vi "DIsco_Main.vi"() -> ()   [LabVIEW 2017]
doc: "DIsco V1.X\n\nDeveloped by Luke P Frash\nLos Alamos National Laboratory"
uses:
  DIsco_Subs.llb/DIsco_Globals.vi
panel:
  out "COM":bool=TRUE
  out "WARN":bool=TRUE
  out "LNK":bool
  out "INIT":bool
  out "AUX":bool
  out "CALL":bool
  in  "Enable Data Saving":bool=TRUE caption="Enable"
  in  "Filename":path=path "C:/ProgramData/Sys_DIsc.lvm"
  out "Date":string
  in  "HistData Empty":bool
  in  "HistData Clear":bool
  out "Recorded Data":string[][](table)
  in  "stop":bool
  in  "Tab Control":enum32{"Valve Positions", "Valve Control Mode"}(tab)
  in  "Valve 4":bool
  in  "Valve 3":bool
  in  "Valve 2":bool
  in  "Valve":bool
  out "VI 1":bool
  out "VI 2":bool
  out "VI 3":bool
  out "VI 4":bool
  in  "Valve 8":bool
  in  "Valve 7":bool
  in  "Valve 6":bool
  in  "Valve 5":bool
  out "VI 5":bool
  out "VI 6":bool
  out "VI 7":bool
  out "VI 8":bool
  in  "SetValves":bool
  in  "Valve 13":bool
  in  "Valve 14":bool
  in  "Valve 15":bool
  in  "Valve 16":bool
  out "VI 13":bool
  out "VI 14":bool
  out "VI 15":bool
  out "VI 16":bool
  in  "Valve 9":bool
  in  "Valve 10":bool
  in  "Valve 11":bool
  in  "Valve 12":bool
  out "VI 9":bool
  out "VI 10":bool
  out "VI 11":bool
  out "VI 12":bool
  in  "SetValves 2":bool
  out "Valve R I":bool
  in  "Set Valve Control":bool
  out "ERR":bool=TRUE
  out "Program":bool
  in  "Track Pump Index":bool=TRUE
  out "F Active":dbl
  out "P Active":dbl
  out "Name of Selected Pump":string
  in  "RenamePump":bool
  in  "Rename":string
  out "CF Ind":bool
  out "CP Ind":bool
  out "CCP Ind":bool
  out "CCF Ind":bool
  in  "CCF":bool
  in  "CCP":bool
  in  "Remote":bool
  in  "Control ID":i32 min=0
  out "Status":string[](array[string])
  out "Pump Type":string
  out "Call ID":i32
  in  "Zero Pres":bool
  out "Letter":string
  in  "Pump Index":i32 min=0 max=4
  out "V Active":dbl
  out "Vol %":u8(slide) scale=0.0..100.0
  in  "Stop":bool
  in  "Run":bool
  in  "CP":bool
  in  "CF":bool
  in  "Pressure Setpoint":dbl min=0.0
  in  "Flow Setpoint":dbl
  in  "SetPress":bool
  in  "SetFlow":bool
  in  "Stop Pumps":bool
  out "Plot1 3":cluster{"X":dbl[], "Y":dbl[]}[](graph) caption="XY Graph"
  in  "X":string="Time"
  in  "Ref":string="log(0)"
  in  "Y6":string
  in  "Y5":string
  in  "Y4":string
  in  "Y3":string
  in  "Y2":string
  in  "Y1":string
  in  "Max_Y 3":dbl=68947.5729
  in  "Min_Y 3":dbl
  in  "Num Points 3":i32=100 min=2 max=10000 step=1
  in  "Max Log":dbl=30.0 min=1e-08 max=1000.0
  in  "Min Log":dbl=1e-06 min=1e-08 max=1000.0
  out "Pump Matrix":string[][](table)
  in  "Tab Control 2":T1(tab)
  in  "Program Edit Table":string[][](table)
  in  "Remove":bool
  in  "AddIt":bool
  in  "Program Selector":i32 min=-1 max=13
  in  "Routine Name":string caption="Program Editor / Importer"
  out "Meaning":string="cSUB PROGRAM : Initiates the pre-set program of NAME."
  out "Active Routine":string="RemoteStartup"
  out "Step":i32
  in  "Set Program":bool
  in  "Reset":bool
  in  "Run Program":bool
  in  "Import CSV":bool
  in  "Export":bool
  out "Countdown":dbl format="%#.1f"
  in  "Pump Index 2":i32 caption="Pump Index" min=0 max=1
  in  "Command":string
  in  "Manual\nExecute":bool
  out "Previous Serial Reply":string
  in  "Append":string caption="Append (eg 13.37)"
  in  "Browse":i32=28 min=0
  out "Description":string
  out "Previous Command":string
  in  "Add Var":bool
  in  "Set Var":bool
  in  "Input Variable (Name=Function)":string
  out "Table Control":string[][](table)
  in  "Add V Index":i32 min=0
  out "Var N":string
  out "Var V":dbl
  in  "E_Add":bool
  out "External Data":dbl[][](array[numeric])
  in  "Import":bool
  in  "External File Path":path=path "C:/Users/299494/Documents/Research/Engineering Design/Programs/DIsco_v1.0/Test Data/Sys_ExtD.lvm"
  in  "E_Col_Name":string
  in  "E_Col_Index":i32
  in  "ExtData Clear":bool
  out "Prog Fetch":i32
  out "Prev Select":i32
  in  "Log Commands":bool=TRUE
  in  "Ask_Auto":bool=TRUE
  in  "Stop Pumps on Exit":bool=TRUE
  in  "Data Call Rate":dbl=1.0 min=0.0001 max=2.0
  in  "Start Time":dbl caption="Reference Date (Time Zero)" format="%#_8g"
  out "Call Execution Time (ms)":u32
  out "Scaling Relationship 3":string="Scaling Factor: 2000*log(WF**-(F+Res))+30000"
  out "Fetch":i32=-1
  out "Heirarchy":string
  out "Passing String":string
  out "Program Errors":string
  out "Running Program":string[][](table)
  out "Brow":i32=28
  out "EXIT":bool
  out "Remote Indicator":bool caption="R/I"
  # "*Units: Min, Days, kPa, mL/min, mL"
  # "Select Pump"
  # "Index"
  # "Letter"
  # "Type"
  # "Setpoint"
  # "Actual Value"
  # "Pump Name"
  # "Pressure (kPa)"
  # "Flow Rate (mL/min)"
  # "Volume (mL)"
  # "Pump Status"
  # "Valve Control"
  # "1"
  # "2"
  # "3"
  # "4"
  # "5"
  # "6"
  # "7"
  # "8"
  # "1"
  # "2"
  # "3"
  # "4"
  # "5"
  # "6"
  # "7"
  # "8"
  # "Plot Settings"
  # "Linear"
  # "log"
  # "Max Linear"
  # "Min Linear"
  # "Max Log"
  # "Min Log"
  # "Points"
  # "Active Routine"
  # "(min)"
  # "Edit Routine"
  # "Selector"
  # "Pump Routine Name"
  # "Manual Command Entry"
  # "Reply to Manual Command"
  # "Input Variable"
  # "Name=[Function] or [Value]"
  # "eg: \"Var1=Var2^2-log(3)/exp(2.32)\""
  # "Add Variable to Data History"
  # "Index"
  # "Name"
  # "Value"
  # "Variable List"
  # "Select CSV Data File to Import"
  # "Add New Column to Data History"
  # "Name"
  # "Col."
  # "Remove All External Data"
  # "Selected External Data"
  # "Data Aquisition Settings"
  # "Hz"
  # "Days"
  # "General Settings"
  # "Log Program Commands"
  # "Ask for Automatic Pump Detection"
  # "Plot Scaling"
  # "Pump Program Parameters"
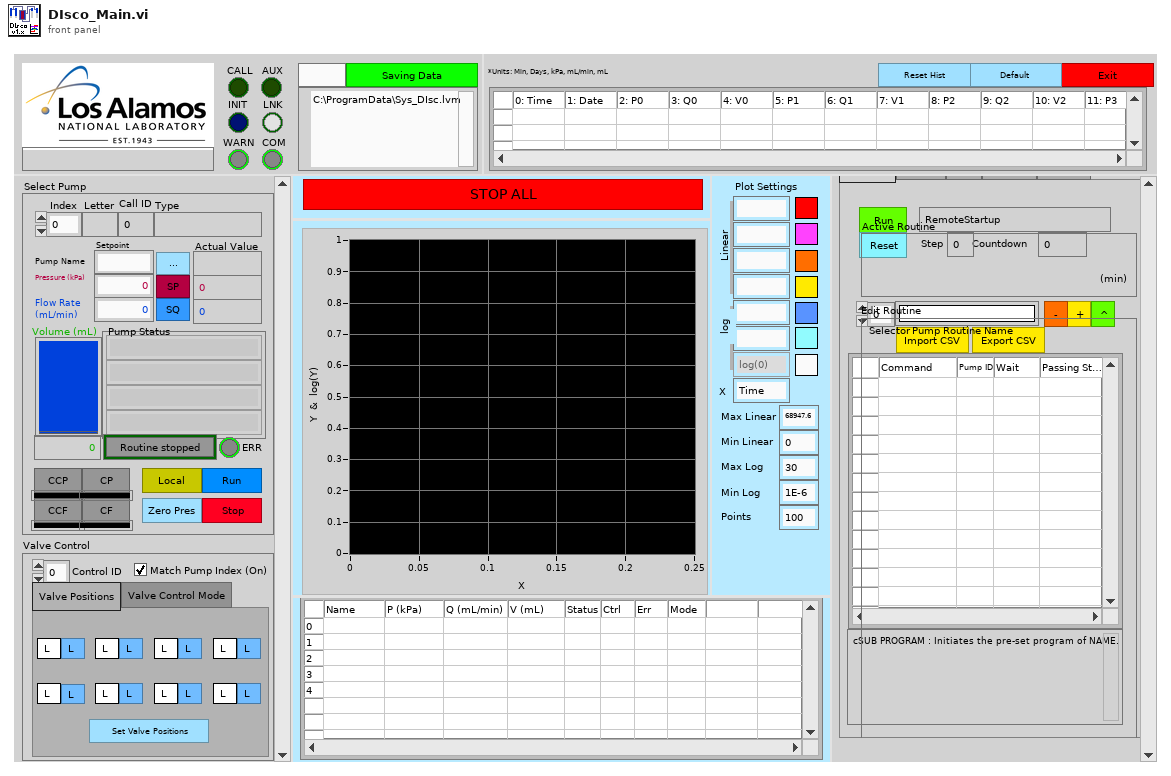
[diagram p1: front panel]
types:
  T1 = enum32{"Routines", "Manual", "Vars", "External", "Settings"}
  T2 = enum8{"Enabled", "Disabled", "Disabled and Grayed Out"}
  T3 = typedef "LVRowAndColumnTypeDef.ctl" = cluster{"Row":i32, "Column":i32}
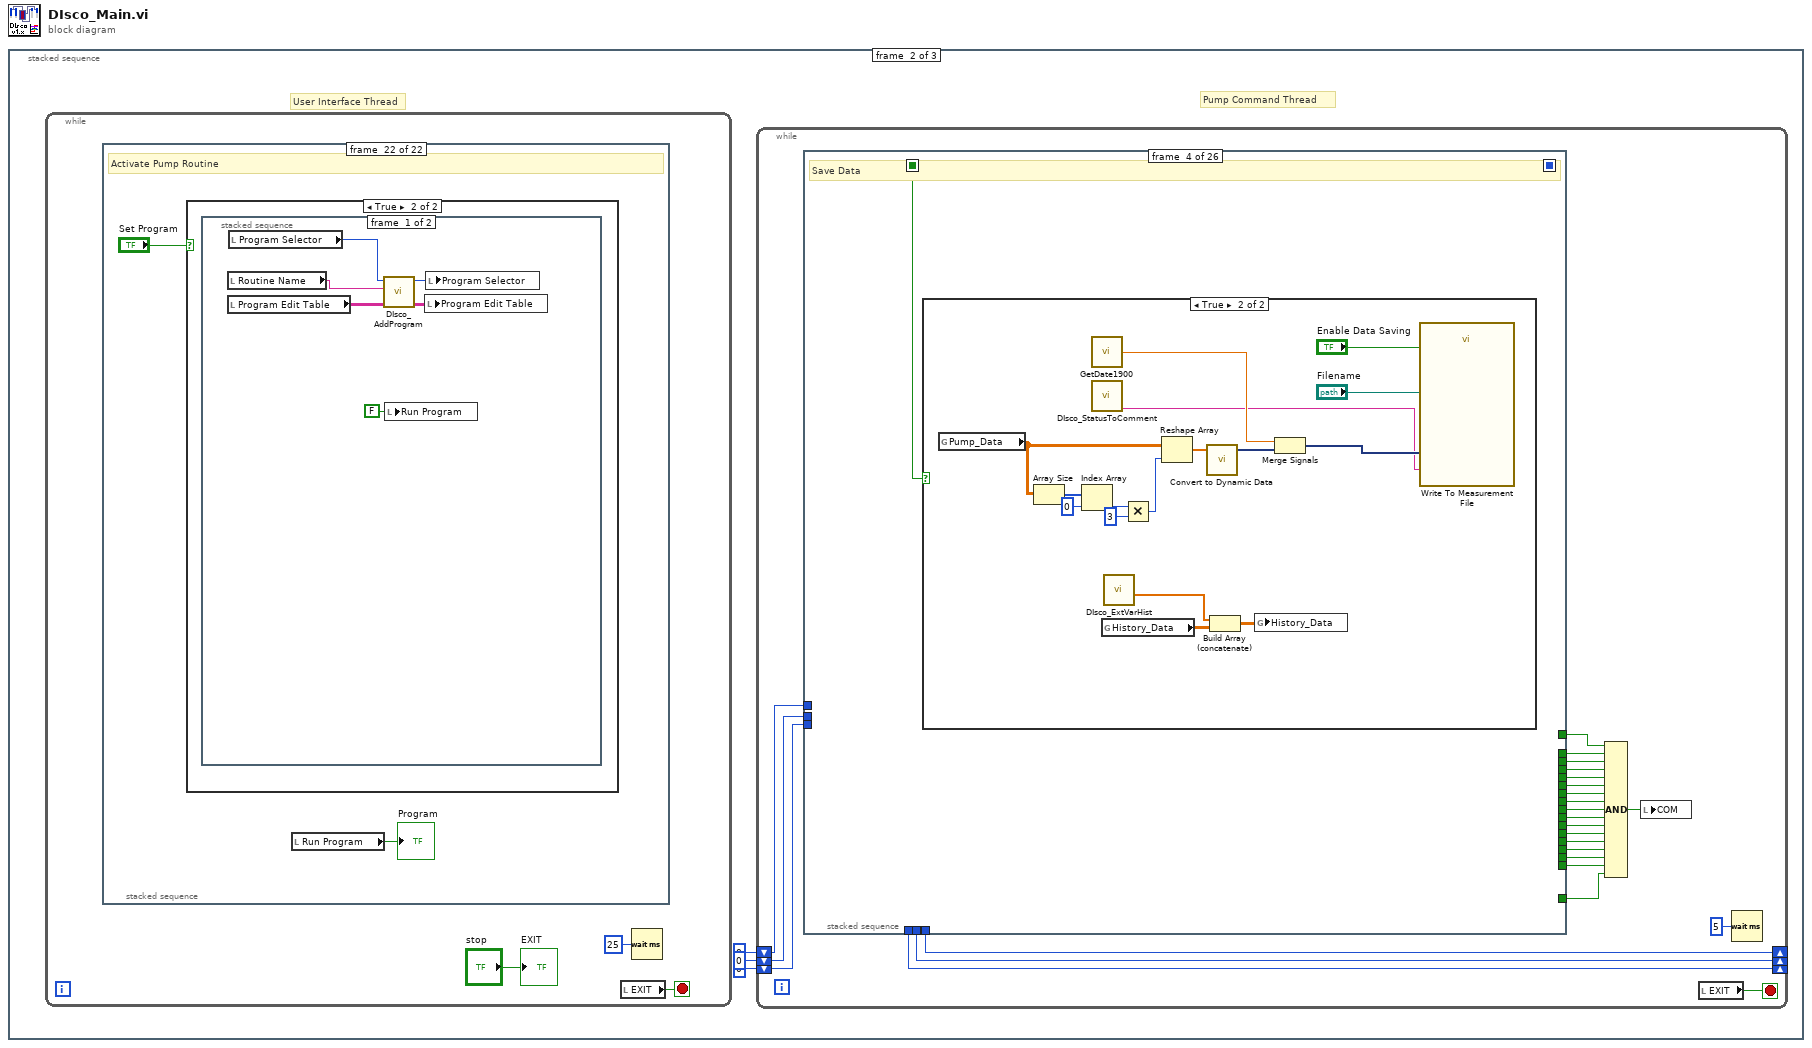
[diagram p0: block diagram]
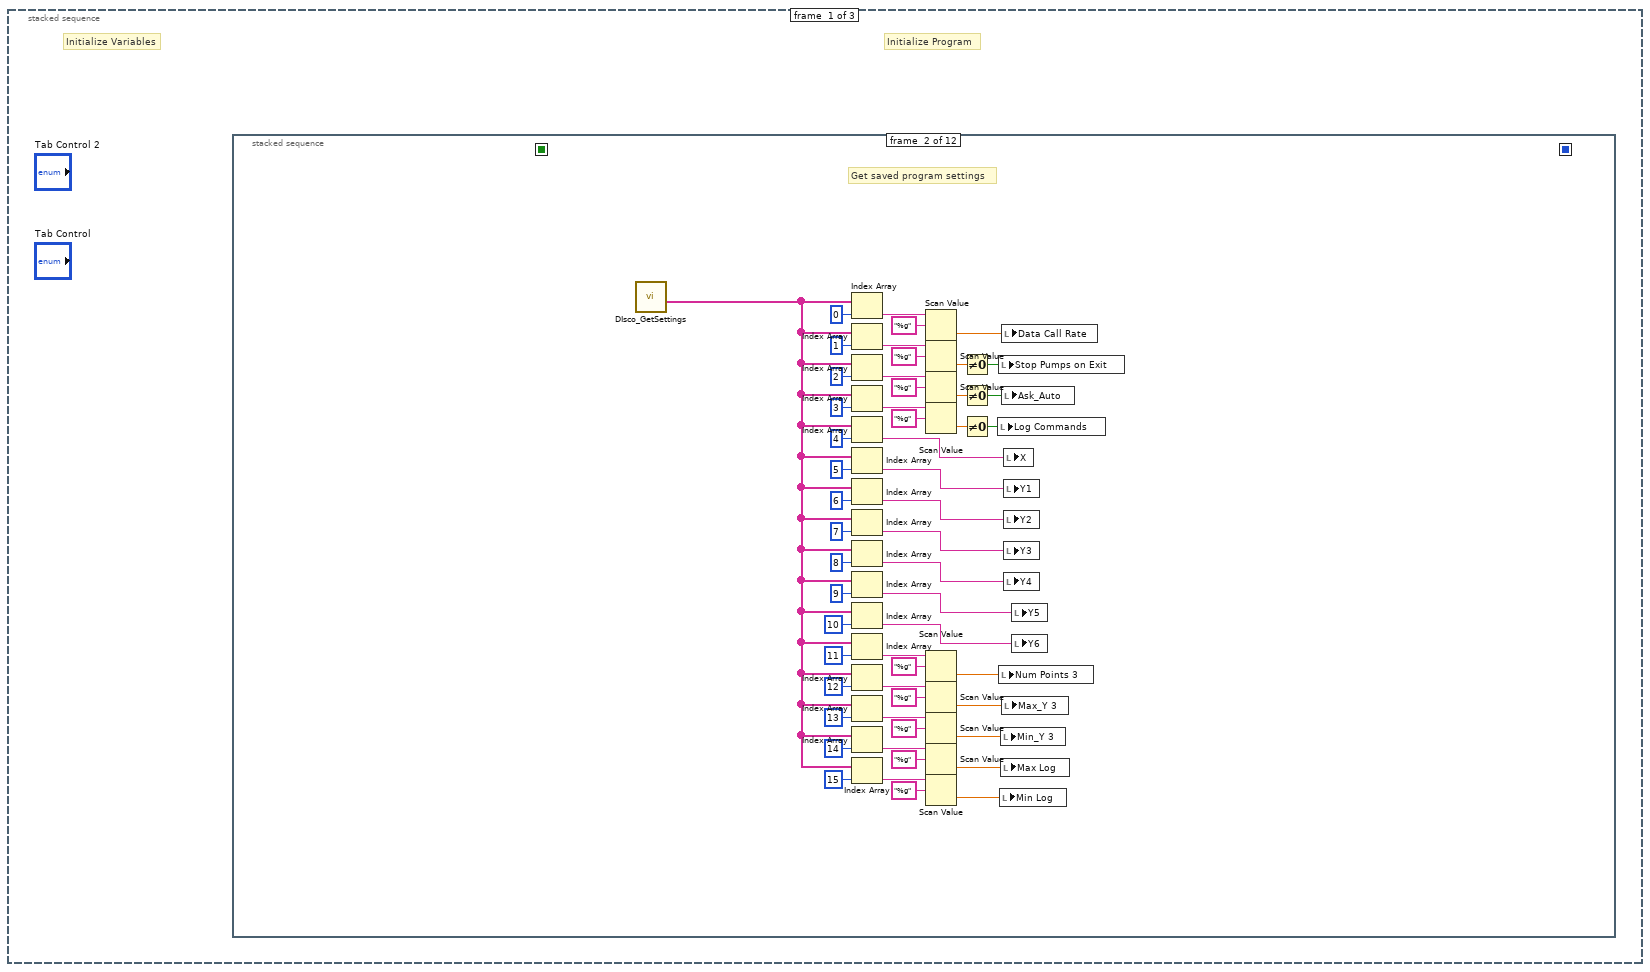
[diagram p2: hidden frame]
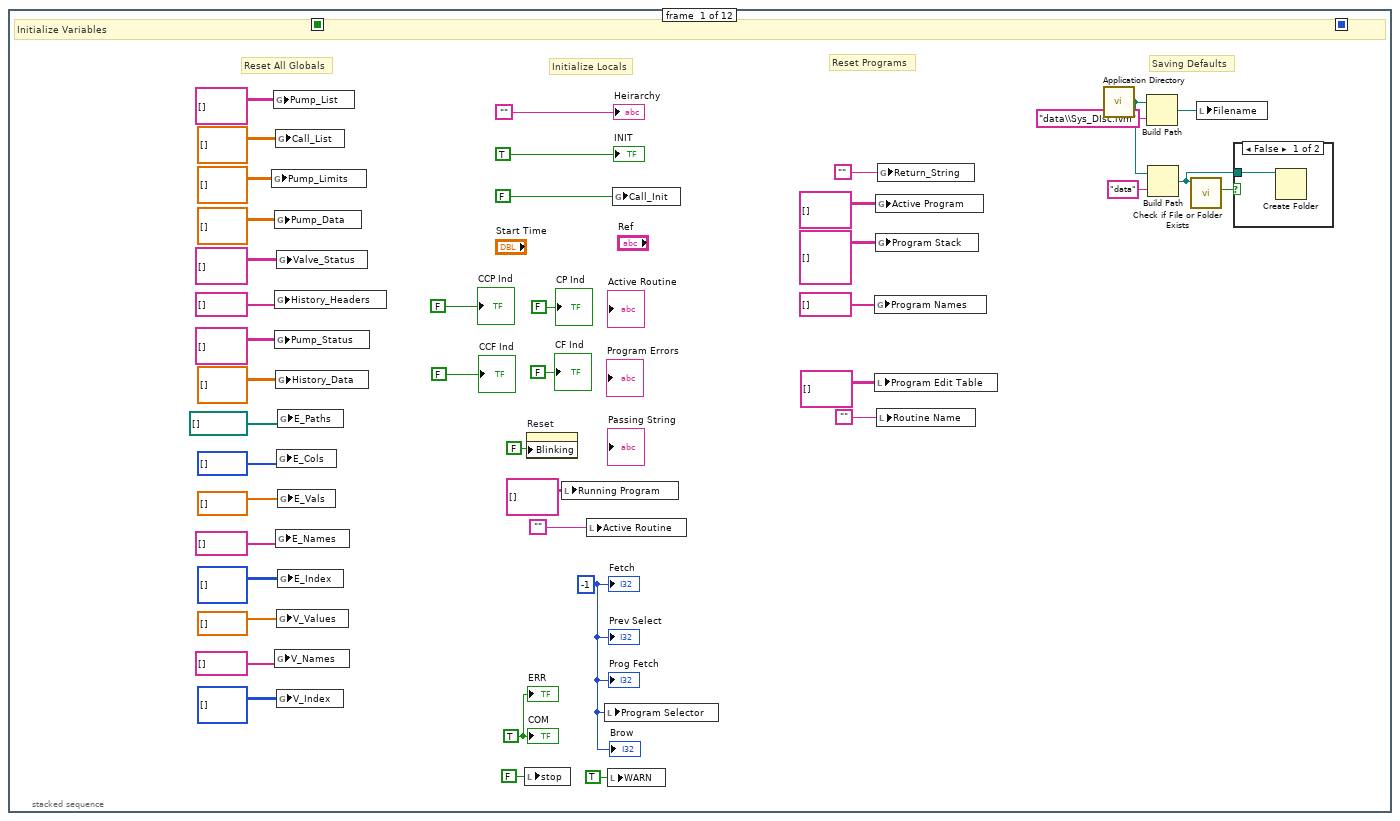
[diagram p3: hidden frame]
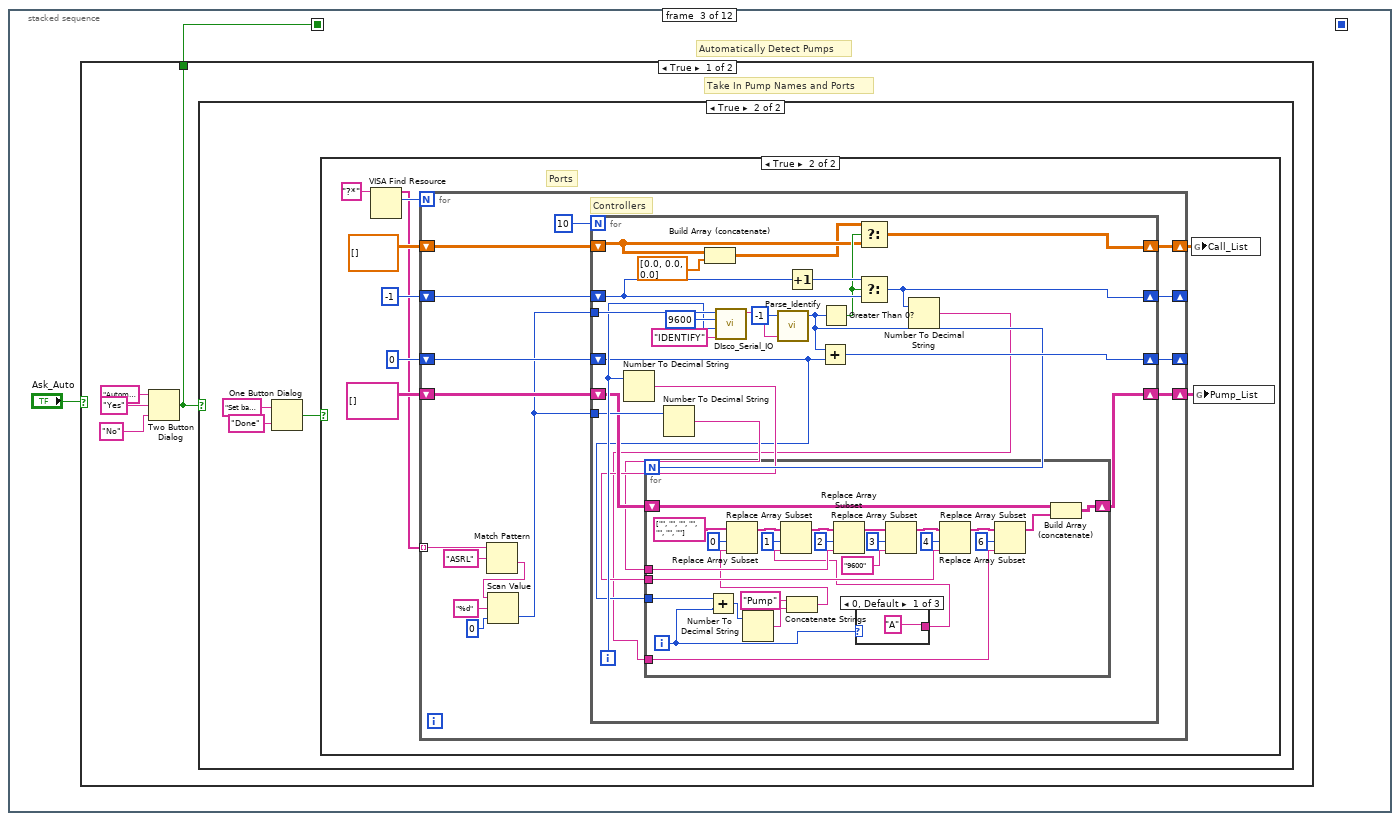
[diagram p5: hidden frame]
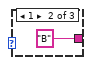
[diagram p8: hidden frame]
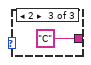
[diagram p9: hidden frame]
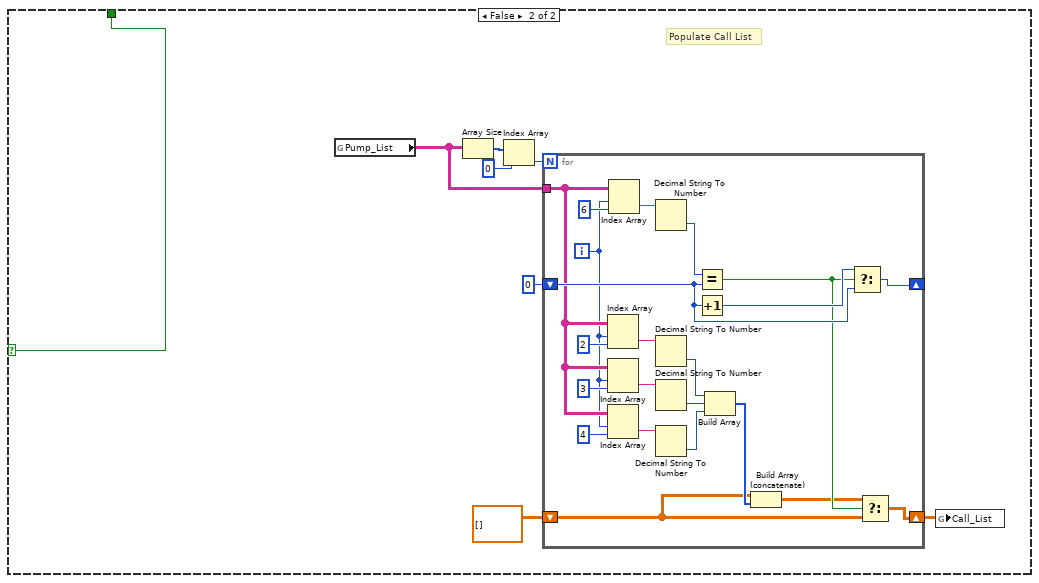
[diagram p10: hidden frame]
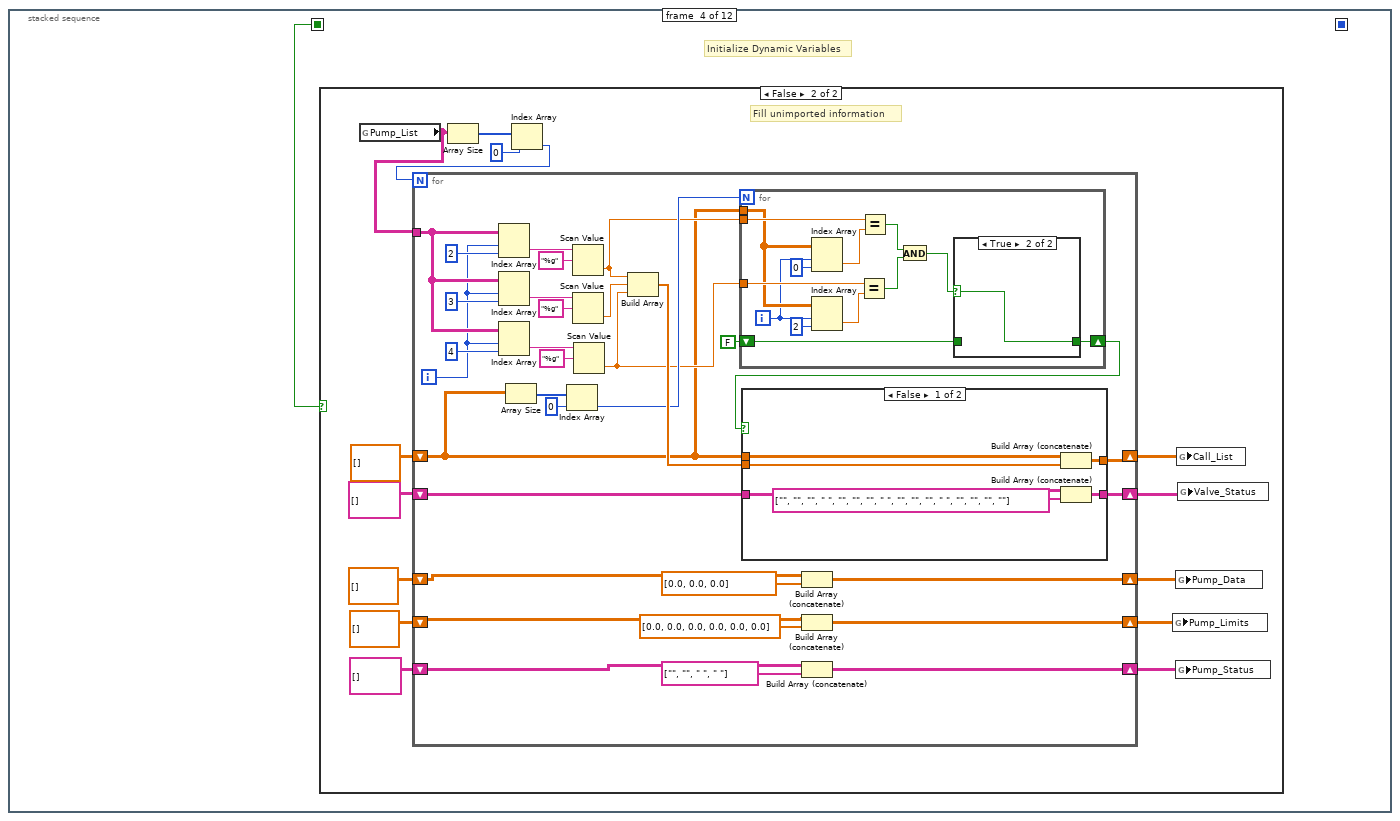
[diagram p11: hidden frame]
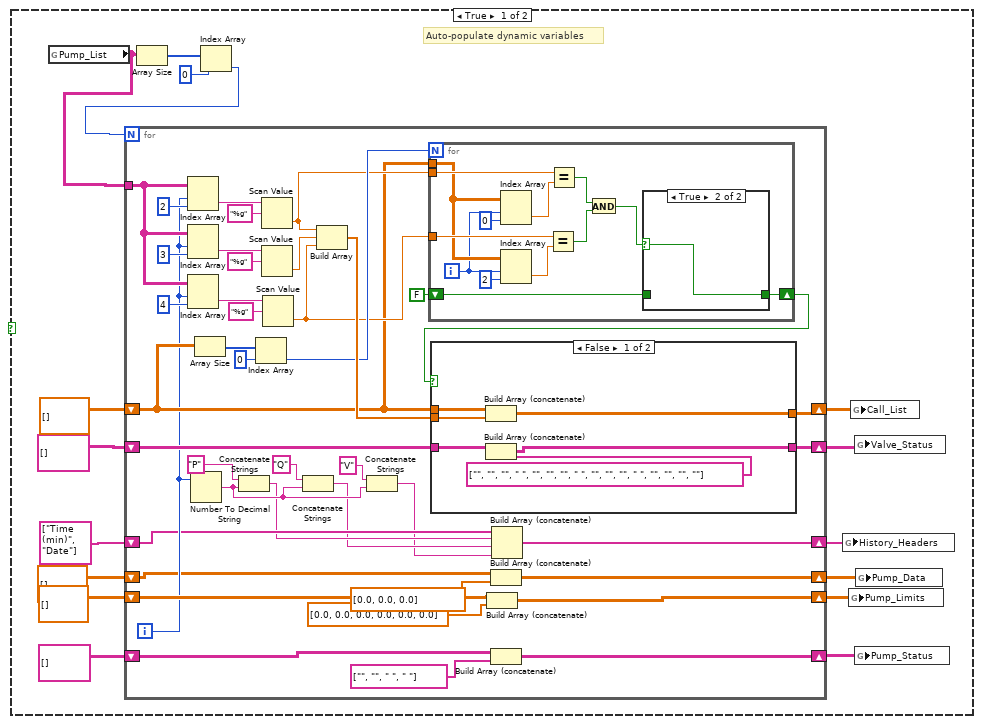
[diagram p12: hidden frame]
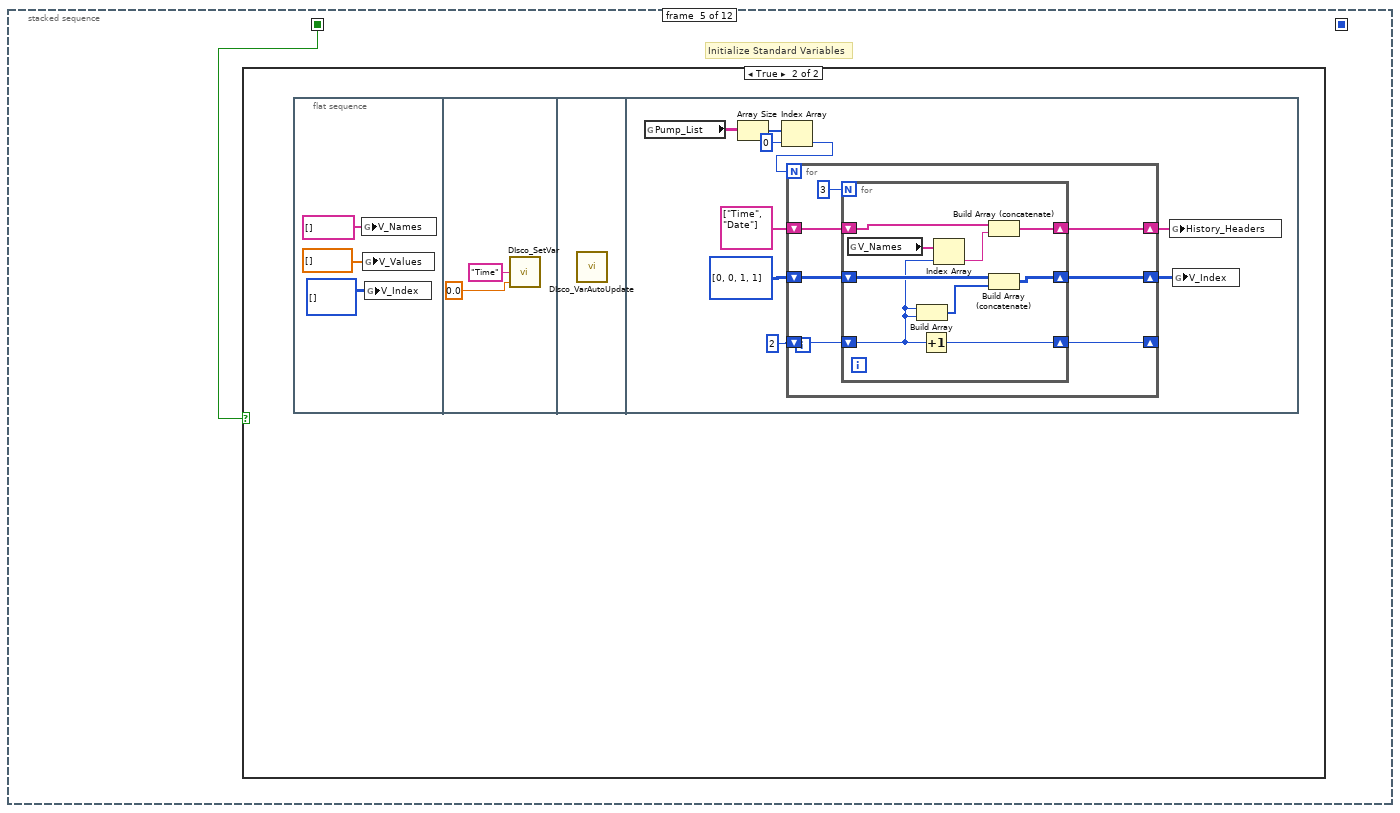
[diagram p17: hidden frame]
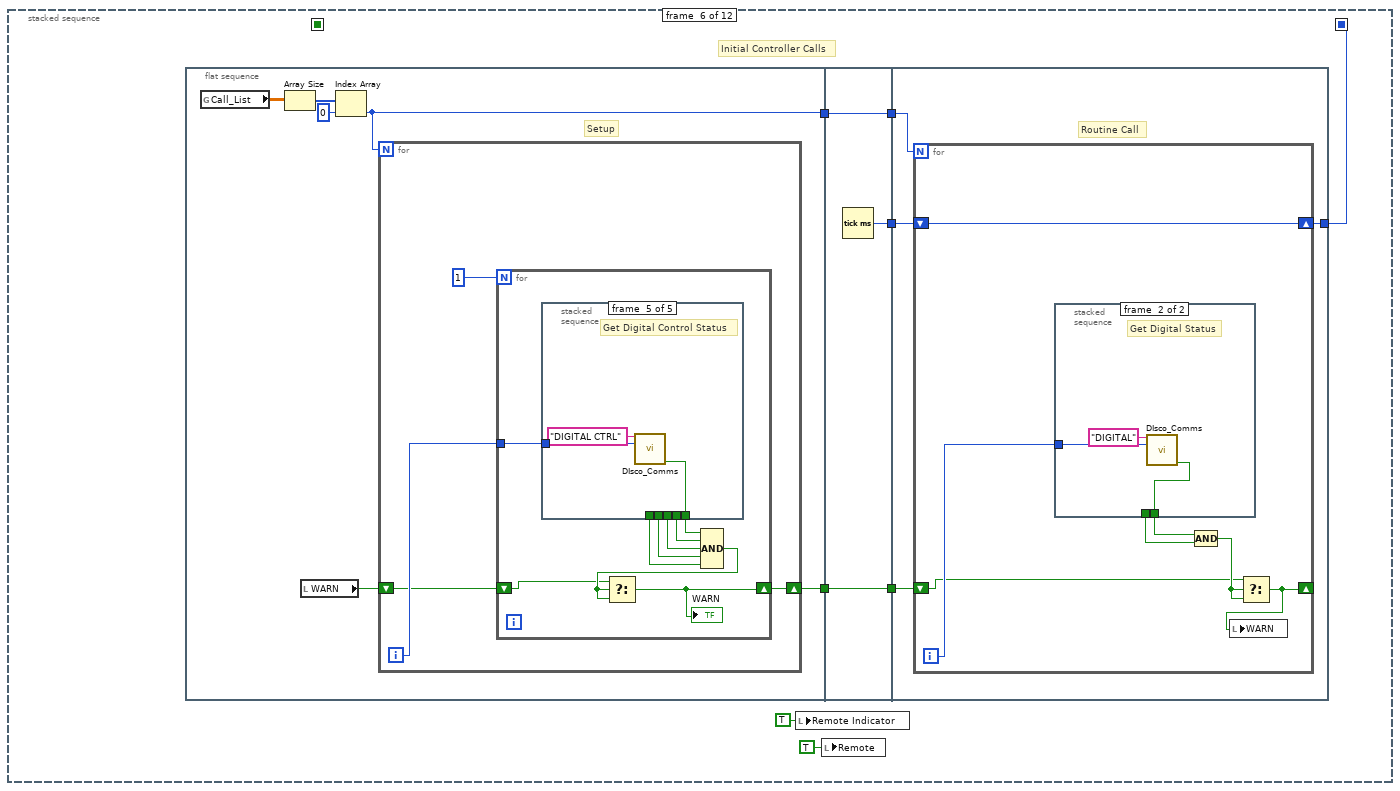
[diagram p19: hidden frame]
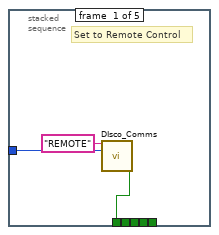
[diagram p20: hidden frame]
diagram:
  n1 = stacked-sequence {
    frame #0 {
      # "Initialize Variables"
      # "Initialize Program"
      n2 = stacked-sequence {
        seq-local: [_ _ w99 _ _ _ _ _ _ _ _ _] -> [_ _ _ w213 w365 _ w460 _ w492 _ _ _]
        seq-local: [_ _ _ _ _ w400 _ _ _ _ _ _] -> [_ _ _ _ _ _ w464 _ _ _ _ _]
        frame #0 {
          w1 = TRUE ("COM")
          w4 = -1 ("Fetch")
          # "Saving Defaults"
          # "Reset Programs"
          # "Initialize Locals"
          # "Reset All Globals"
          # "Initialize Variables"
          n3 = global write "DIsco_Globals.vi" "Pump_Limits"(dbl[][] [] ("Pump_Limits")) -> ()
          n4 = global write "DIsco_Globals.vi" "Pump_List"(string[][] [] ("Valve_Status")) -> ()
          n5 = global write "DIsco_Globals.vi" "Pump_Data"(dbl[][] [] ("Pump_Limits")) -> ()
          n6 = global write "DIsco_Globals.vi" "History_Headers"(string[] [] ("Valve_Status")) -> ()
          n7 = global write "DIsco_Globals.vi" "Pump_Status"(string[][] [] ("Valve_Status")) -> ()
          n8 = global write "DIsco_Globals.vi" "V_Names"(string[] [] ("Valve_Status")) -> ()
          n9 = global write "DIsco_Globals.vi" "Call_List"(dbl[][] [] ("Call_List")) -> ()
          n10 = global write "DIsco_Globals.vi" "History_Data"(dbl[][] [] ("History_Data")) -> ()
          n11 = global write "DIsco_Globals.vi" "E_Names"(string[] [] ("Valve_Status")) -> ()
          n12 = global write "DIsco_Globals.vi" "Valve_Status"(string[][] [] ("Valve_Status")) -> ()
          n13 = global write "DIsco_Globals.vi" "E_Cols"(i32[] [] ("E_Cols")) -> ()
          n14 = global write "DIsco_Globals.vi" "V_Values"(dbl[] [] ("History_Data")) -> ()
          n15 = global write "DIsco_Globals.vi" "V_Index"(i32[][] [] ("E_Cols")) -> ()
          n16 = global write "DIsco_Globals.vi" "E_Paths"(path[] [] ("E_Paths")) -> ()
          n17 = global write "DIsco_Globals.vi" "E_Vals"(dbl[] [] ("History_Data")) -> ()
          n18 = global write "DIsco_Globals.vi" "E_Index"(i32[][] [] ("E_Cols")) -> ()
          n19 = local write "stop"(FALSE ("stop")) -> ()
          n20 = property on="Reset" class="Bool (strict)"("Blinking"=FALSE) -> ()  [unwired: 2 in, 2 out]
          n21 = local write "Running Program"(string[][] [] ("Running Program")) -> ()
          n22 = local write "Active Routine"("") -> ()
          n23 = local write "Program Selector"(w4) -> ()
          n24 = local write "WARN"(TRUE ("WARN")) -> ()
          n25 = global write "DIsco_Globals.vi" "Call_Init"(FALSE ("Call_Init")) -> ()
          n26 = global write "DIsco_Globals.vi" "Program Names"(string[] [] ("Valve_Status")) -> ()
          n27 = local write "Program Edit Table"(string[][] [] ("Program Edit Table")) -> ()
          n28 = global write "DIsco_Globals.vi" "Active Program"(string[][] [] ("Valve_Status")) -> ()
          n29 = global write "DIsco_Globals.vi" "Program Stack"(string[][][] [] ("Valve_Status")) -> ()
          n30 = local write "Routine Name"("") -> ()
          n31 = global write "DIsco_Globals.vi" "Return_String"("") -> ()
          n32 = call <vilib>:"Application Directory.vi"() -> ("Application Directory"=w8:path)
          n33 = Build Path(base path=w8, name or relative path="data\\Sys_DIsc.lvm") -> (appended path=w22:path)
          n34 = Build Path(base path=w8, name or relative path="data") -> (appended path=w5:path)
          n35 = call <vilib>:"Check if File or Folder Exists.vi"("path"=w5) -> ("file or folder exists?"=w6:bool)  [unwired: 8 in, 2 out]
          n36 = local write "Filename"(w22) -> ()
          n37 = case shown="False" w6 {
            tunnel: w5 -> [w43 _]
            frame False {
              n38 = Create Folder(path (use dialog)=w43) -> ()  [unwired: 2 in, 3 out]
            }
            frame True {
            }
          }
          "INIT" <- TRUE ("INIT")
          "Heirarchy" <- ""
          "Fetch" <- w4
          "CP Ind" <- FALSE ("CCP Ind")
          "CF Ind" <- FALSE ("CCP Ind")
          "CCP Ind" <- FALSE ("CCP Ind")
          "CCF Ind" <- FALSE ("CCF Ind")
          "Prev Select" <- w4
          "Prog Fetch" <- w4
          "Brow" <- w4
          "COM" <- w1
          "ERR" <- w1
        }
        frame #1 {
          # "Get saved program settings"
          n39 = call "DIsco_GetSettings.vi"() -> ("General Settings"=w56:string[])  [unwired: 11 in]
          n40 = Index Array(array=w56, index=0) -> (element=w96:string)
          n41 = Index Array(array=w56, index=1) -> (element=w93:string)
          n42 = Index Array(array=w56, index=2) -> (element=w89:string)
          n43 = Index Array(array=w56, index=3) -> (element=w85:string)
          n44 = Index Array(array=w56, index=4) -> (element=w44:string)
          n45 = Index Array(array=w56, index=5) -> (element=w50:string)
          n46 = Index Array(array=w56, index=6) -> (element=w49:string)
          n47 = Index Array(array=w56, index=7) -> (element=w48:string)
          n48 = Index Array(array=w56, index=8) -> (element=w47:string)
          n49 = Index Array(array=w56, index=9) -> (element=w46:string)
          n50 = Index Array(array=w56, index=10) -> (element=w45:string)
          n51 = Index Array(array=w56, index=11) -> (element=w70:string)
          n52 = Index Array(array=w56, index=12) -> (element=w67:string)
          n53 = Index Array(array=w56, index=13) -> (element=w64:string)
          n54 = Index Array(array=w56, index=14) -> (element=w61:string)
          n55 = Index Array(array=w56, index=15) -> (element=w58:string)
          n56 = Scan Value(string=w96, format string="%g") -> (value=w82:dbl)  [unwired: 1 in, 1 out]
          n57 = Scan Value(string=w93, format string="%g") -> (value=w91:dbl)  [unwired: 1 in, 1 out]
          n58 = Scan Value(string=w89, format string="%g") -> (value=w87:dbl)  [unwired: 1 in, 1 out]
          n59 = Scan Value(string=w85, format string="%g") -> (value=w83:dbl)  [unwired: 1 in, 1 out]
          n60 = Scan Value(string=w70, format string="%g") -> (value=w55:dbl)  [unwired: 1 in, 1 out]
          n61 = Scan Value(string=w67, format string="%g") -> (value=w54:dbl)  [unwired: 1 in, 1 out]
          n62 = Scan Value(string=w64, format string="%g") -> (value=w53:dbl)  [unwired: 1 in, 1 out]
          n63 = Scan Value(string=w61, format string="%g") -> (value=w52:dbl)  [unwired: 1 in, 1 out]
          n64 = Scan Value(string=w58, format string="%g") -> (value=w51:dbl)  [unwired: 1 in, 1 out]
          n65 = Not Equal To 0?(x=w91) -> (x != 0?=w81:bool)
          n66 = Not Equal To 0?(x=w87) -> (x != 0?=w80:bool)
          n67 = Not Equal To 0?(x=w83) -> (x != 0?=w79:bool)
          n68 = local write "Log Commands"(w79) -> ()
          n69 = local write "Stop Pumps on Exit"(w81) -> ()
          n70 = local write "Num Points 3"(w55) -> ()
          n71 = local write "Min Log"(w51) -> ()
          n72 = local write "Min_Y 3"(w53) -> ()
          n73 = local write "Max Log"(w52) -> ()
          n74 = local write "Data Call Rate"(w82) -> ()
          n75 = local write "Ask_Auto"(w80) -> ()
          n76 = local write "Max_Y 3"(w54) -> ()
          n77 = local write "X"(w44) -> ()
          n78 = local write "Y1"(w50) -> ()
          n79 = local write "Y2"(w49) -> ()
          n80 = local write "Y3"(w48) -> ()
          n81 = local write "Y4"(w47) -> ()
          n82 = local write "Y5"(w46) -> ()
          n83 = local write "Y6"(w45) -> ()
        }
        frame #2 {
          # "Automatically Detect Pumps"
          n84 = case shown="True" "Ask_Auto" {
            selector: "Ask_Auto" -> [_ w185]
            tunnel: [w100 w185] -> w99
            frame True {
              # "Take In Pump Names and Ports"
              n85 = Two Button Dialog(message="Automatically detect attached pumps?", 1:"No" ("F button name (\"Cancel\")"), 2:"Yes" ("T button name (\"OK\")")) -> (T button?=w100:bool)
              n86 = case shown="True" w100 {
                frame False {
                }
                frame True {
                  n87 = One Button Dialog(message="Set baud rate on all controllers to 9600", button name ("OK")="Done") -> (true=w104:bool)
                  n88 = case shown="True" w104 {
                    frame False {
                    }
                    frame True {
                      # "Ports"
                      n89 = VISA Find Resource(11:"?*" ("expression (\"?*\")")) -> (2:w108:u32, 3:w107:string[])  [unwired: 2 in, 1 out]
                      n90 = for {
                        N: w108 -> [_]
                        shift-right: [w129] -> _
                        shift-left: 0 ("nCommand") -> [w130]
                        shift-right: [w126] -> _
                        shift-left: -1 ("nCommand") -> [w127]
                        shift-right: [w124] -> w112
                        shift-left: string[][] [] ("Pump_List") -> [w125]
                        shift-right: [w123] -> w110
                        shift-left: dbl[][] [] ("Call_List") -> [w122]
                        tunnel: w107 -> [w121] mode=indexing
                        # "Controllers"
                        n91 = Match Pattern(string=w121, regular expression="ASRL") -> (after substring=w119:string)  [unwired: 1 in, 3 out]
                        n92 = Scan Value(string=w119, format string="%d", default (0 dbl)=0) -> (value=w116:i32)  [unwired: 1 out]
                        n93 = for {
                          N: 10 -> [_]
                          shift-right: [w149] -> w129
                          shift-left: w130 -> [w139]
                          tunnel: w116 -> [w150]
                          shift-right: [w138] -> w126
                          shift-left: w127 -> [w147]
                          shift-right: [w142] -> w124
                          shift-left: w125 -> [w144]
                          tunnel: w116 -> [w145]
                          shift-right: [w133] -> w123
                          shift-left: w122 -> [w135]
                          i -> [w146]
                          n94 = Number To Decimal String(number=w146) -> (decimal integer string=w141:string)  [unwired: 1 in]
                          n95 = Number To Decimal String(number=w145) -> (decimal integer string=w140:string)  [unwired: 1 in]
                          n96 = Build Array (concatenate)(w135, dbl[] [0.0, 0.0, 0.0] ("Call_List")) -> (w134:dbl[][])
                          n97 = call "DIsco_Serial_IO.vi"("Pump Command"="IDENTIFY", "Controller ID"=w146, "Baud Rate"=9600, "Port"=w150) -> ("Reply"=w153:string)  [unwired: 6 in, 1 out]
                          n98 = call "Parse_Identify.vi"("Pump Info"=w153, "Call Index"=-1) -> ("Number of Pumps"=w143:i32)  [unwired: 1 in, 2 out]
                          n99 = Increment(x=w147) -> (x+1=w148:i32)
                          n100 = Add(x=w143, y=w139) -> (x+y=w149:i32)
                          n101 = Greater Than 0?(x=w143) -> (x > 0?=w136:bool)
                          n102 = Select(t=w134, s=w136, f=w135) -> (s? t:f=w133:dbl[][])
                          n103 = Select(t=w148, s=w136, f=w147) -> (s? t:f=w138:i32)
                          n104 = Number To Decimal String(number=w138) -> (decimal integer string=w137:string)  [unwired: 1 in]
                          n105 = for {
                            N: w143 -> [_]
                            shift-right: [w165] -> w142
                            shift-left: w144 -> [w166]
                            tunnel: w141 -> [w163]
                            tunnel: w140 -> [w162]
                            tunnel: w139 -> [w159]
                            tunnel: w137 -> [w155]
                            i -> [w154]
                            n106 = Add(x=w159, y=w154) -> (x+y=w158:i32)
                            n107 = Number To Decimal String(number=w158) -> (decimal integer string=w161:string)  [unwired: 1 in]
                            n108 = Concatenate Strings("Pump" ("string"), w161) -> (w157:string)
                            n109 = Replace Array Subset(array=string[] ["", "", "", "", "", "", ""] ("Array"), new element=w157, index=0) -> (w172:string[])
                            n110 = case shown="0, Default" w154 {
                              tunnel: ["A" ("new element/subarray") "B" ("new element/subarray") "C" ("new element/subarray")] -> w156
                              frame 0, Default {
                              }
                              frame 1 {
                              }
                              frame 2 {
                              }
                            }
                            n111 = Replace Array Subset(array=w172, new element=w156, index=1) -> (w171:string[])
                            n112 = Replace Array Subset(array=w171, new element=w162, index=2) -> (w170:string[])
                            n113 = Replace Array Subset(array=w170, new element="9600" ("new element/subarray"), index=3) -> (w169:string[])
                            n114 = Replace Array Subset(array=w169, new element=w163, index=4) -> (w168:string[])
                            n115 = Replace Array Subset(array=w168, new element=w155, index=6) -> (w167:string[])
                            n116 = Build Array (concatenate)(w166, w167) -> (w165:string[][])
                          }
                        }
                      }
                      n117 = global write "DIsco_Globals.vi" "Call_List"(w110) -> ()
                      n118 = global write "DIsco_Globals.vi" "Pump_List"(w112) -> ()
                    }
                  }
                }
              }
            }
            frame False {
              # "Populate Call List"
              n119 = global read "DIsco_Globals.vi" "Pump_List"() -> (w184:string[][])
              n120 = Array Size(array=w184) -> (size(s)=w188:i32[])
              n121 = Index Array(array=w188, index=0) -> (element=w186:i32)
              n122 = for {
                N: w186 -> [_]
                shift-right: [w191] -> w189
                shift-left: dbl[][] [] ("Call_List") -> [w192]
                tunnel: w184 -> [w203]
                shift-right: [w207] -> _
                shift-left: 0 ("index") -> [w208]
                i -> [w202]
                n123 = Index Array(array=w203, index (row)=w202, index (col)=2 ("disabled index (col)")) -> (element=w201:string)
                n124 = Index Array(array=w203, index (row)=w202, index (col)=3 ("disabled index (col)")) -> (element=w200:string)
                n125 = Index Array(array=w203, index (row)=w202, index (col)=4 ("disabled index (col)")) -> (element=w199:string)
                n126 = Index Array(array=w203, index (row)=w202, index (col)=6 ("disabled index (col)")) -> (element=w211:string)
                n127 = Decimal String To Number(string=w211) -> (number=w210:i32)  [unwired: 2 in, 1 out]
                n128 = Decimal String To Number(string=w201) -> (number=w198:i32)  [unwired: 2 in, 1 out]
                n129 = Decimal String To Number(string=w200) -> (number=w197:i32)  [unwired: 2 in, 1 out]
                n130 = Decimal String To Number(string=w199) -> (number=w196:i32)  [unwired: 2 in, 1 out]
                n131 = Equal?(x=w210, y=w208) -> (x = y?=w195:bool)
                n132 = Increment(x=w208) -> (x+1=w209:i32)
                n133 = Build Array(w198, w197, w196) -> (w194:i32[])
                n134 = Build Array (concatenate)(w192, w194) -> (w193:dbl[][])
                n135 = Select(t=w209, s=w195, f=w208) -> (s? t:f=w207:i32)
                n136 = Select(t=w193, s=w195, f=w192) -> (s? t:f=w191:dbl[][])
              }
              n137 = global write "DIsco_Globals.vi" "Call_List"(w189) -> ()
            }
          }
        }
        frame #3 {
          # "Initialize Dynamic Variables"
          n138 = case shown="False" w213 {
            frame True {
              # "Auto-populate dynamic variables"
              n139 = global read "DIsco_Globals.vi" "Pump_List"() -> (w219:string[][])
              n140 = Array Size(array=w219) -> (size(s)=w229:i32[])
              n141 = Index Array(array=w229, index=0) -> (element=w218:i32)
              n142 = for {
                N: w218 -> [_]
                shift-right: [w265] -> w226
                shift-left: dbl[][] [] ("Call_List") -> [w247]
                shift-right: [w266] -> w224
                shift-left: dbl[][] [] ("Call_List") -> [w267]
                tunnel: w219 -> [w248]
                shift-right: [w244] -> w222
                shift-left: string[][] [] ("Valve_Status") -> [w245]
                shift-right: [w256] -> w220
                shift-left: dbl[][] [] ("Call_List") -> [w241]
                shift-right: [w242] -> w216
                shift-left: string[] ["Time (min)", "Date"] ("Valve_Status") -> [w240]
                shift-right: [w230] -> w215
                shift-left: string[][] [] ("Valve_Status") -> [w231]
                i -> [w243]
                n143 = Index Array(array=w248, index (row)=w243, index (col)=2 ("disabled index (col)")) -> (element=w264:string)
                n144 = Index Array(array=w248, index (row)=w243, index (col)=3 ("disabled index (col)")) -> (element=w263:string)
                n145 = Index Array(array=w248, index (row)=w243, index (col)=4 ("disabled index (col)")) -> (element=w262:string)
                n146 = Number To Decimal String(number=w243) -> (decimal integer string=w236:string)  [unwired: 1 in]
                n147 = Array Size(array=w247) -> (size(s)=w254:i32[])
                n148 = Concatenate Strings("P" ("format string"), w236) -> (w235:string)
                n149 = Index Array(array=w254, index=0) -> (element=w252:i32)
                n150 = Scan Value(string=w264, format string="%g") -> (value=w250:dbl)  [unwired: 1 in, 1 out]
                n151 = Scan Value(string=w263, format string="%g") -> (value=w261:dbl)  [unwired: 1 in, 1 out]
                n152 = Scan Value(string=w262, format string="%g") -> (value=w249:dbl)  [unwired: 1 in, 1 out]
                n153 = Concatenate Strings("Q" ("format string"), w236) -> (w234:string)
                n154 = Build Array(w250, w261, w249) -> (w257:dbl[])
                n155 = Concatenate Strings("V" ("format string"), w236) -> (w233:string)
                n156 = for {
                  N: w252 -> [_]
                  shift-right: [w273] -> w246
                  shift-left: FALSE -> [w272]
                  tunnel: w250 -> [w282]
                  tunnel: w249 -> [w281]
                  tunnel: w247 -> [w279]
                  i -> [w277]
                  n157 = Index Array(array=w279, index (row)=w277, index (col)=0 ("index")) -> (element=w276:dbl)
                  n158 = Index Array(array=w279, index (row)=w277, index (col)=2 ("index")) -> (element=w275:dbl)
                  n159 = Equal?(x=w281, y=w275) -> (x = y?=w283:bool)
                  n160 = Equal?(x=w282, y=w276) -> (x = y?=w284:bool)
                  n161 = And(x=w284, y=w283) -> (x .and. y?=w274:bool)
                  n162 = case shown="True" w274 {
                    selector: w274 -> [_ w286]
                    tunnel: [w285 w286] -> w273
                    tunnel: w272 -> [w285 _]
                    frame False {
                    }
                    frame True {
                    }
                  }
                }
                n163 = case shown="False" w246 {
                  tunnel: w247 -> [w292 w294]
                  tunnel: [w291 w294] -> w265
                  tunnel: w257 -> [w290 _]
                  tunnel: w245 -> [w289 w293]
                  tunnel: [w288 w293] -> w244
                  frame False {
                    n164 = Build Array (concatenate)(w292, w290) -> (w291:dbl[][])
                    n165 = Build Array (concatenate)(w289, string[] ["", "", "", " ", "", "", "", " ", "", "", "", " ", "", "", "", ""] ("Valve_Status")) -> (w288:string[][])
                  }
                  frame True {
                  }
                }
                n166 = Build Array (concatenate)(w267, dbl[] [0.0, 0.0, 0.0, 0.0, 0.0, 0.0] ("Call_List")) -> (w266:dbl[][])
                n167 = Build Array (concatenate)(w241, dbl[] [0.0, 0.0, 0.0] ("Call_List")) -> (w256:dbl[][])
                n168 = Build Array (concatenate)(w231, string[] ["", "", " ", " "] ("Valve_Status")) -> (w230:string[][])
                n169 = Build Array (concatenate)(w240, w235, w234, w233) -> (w242:string[])
              }
              n170 = global write "DIsco_Globals.vi" "History_Headers"(w216) -> ()
              n171 = global write "DIsco_Globals.vi" "Pump_Limits"(w224) -> ()
              n172 = global write "DIsco_Globals.vi" "Call_List"(w226) -> ()
              n173 = global write "DIsco_Globals.vi" "Valve_Status"(w222) -> ()
              n174 = global write "DIsco_Globals.vi" "Pump_Status"(w215) -> ()
              n175 = global write "DIsco_Globals.vi" "Pump_Data"(w220) -> ()
            }
            frame False {
              # "Fill unimported information"
              n176 = global read "DIsco_Globals.vi" "Pump_List"() -> (w298:string[][])
              n177 = Array Size(array=w298) -> (size(s)=w308:i32[])
              n178 = Index Array(array=w308, index=0) -> (element=w297:i32)
              n179 = for {
                N: w297 -> [_]
                shift-right: [w336] -> w305
                shift-left: dbl[][] [] ("Call_List") -> [w318]
                shift-right: [w337] -> w303
                shift-left: dbl[][] [] ("Call_List") -> [w309]
                tunnel: w298 -> [w319]
                shift-right: [w315] -> w301
                shift-left: string[][] [] ("Valve_Status") -> [w316]
                shift-right: [w327] -> w299
                shift-left: dbl[][] [] ("Call_List") -> [w313]
                shift-right: [w310] -> w296
                shift-left: string[][] [] ("Valve_Status") -> [w311]
                i -> [w314]
                n180 = Index Array(array=w319, index (row)=w314, index (col)=2 ("disabled index (col)")) -> (element=w335:string)
                n181 = Index Array(array=w319, index (row)=w314, index (col)=3 ("disabled index (col)")) -> (element=w334:string)
                n182 = Index Array(array=w319, index (row)=w314, index (col)=4 ("disabled index (col)")) -> (element=w333:string)
                n183 = Array Size(array=w318) -> (size(s)=w325:i32[])
                n184 = Index Array(array=w325, index=0) -> (element=w323:i32)
                n185 = Scan Value(string=w335, format string="%g") -> (value=w321:dbl)  [unwired: 1 in, 1 out]
                n186 = Scan Value(string=w334, format string="%g") -> (value=w332:dbl)  [unwired: 1 in, 1 out]
                n187 = Scan Value(string=w333, format string="%g") -> (value=w320:dbl)  [unwired: 1 in, 1 out]
                n188 = Build Array(w321, w332, w320) -> (w328:dbl[])
                n189 = for {
                  N: w323 -> [_]
                  shift-right: [w343] -> w317
                  shift-left: FALSE -> [w342]
                  tunnel: w321 -> [w352]
                  tunnel: w320 -> [w351]
                  tunnel: w318 -> [w349]
                  i -> [w347]
                  n190 = Index Array(array=w349, index (row)=w347, index (col)=0 ("index")) -> (element=w346:dbl)
                  n191 = Index Array(array=w349, index (row)=w347, index (col)=2 ("index")) -> (element=w345:dbl)
                  n192 = Equal?(x=w351, y=w345) -> (x = y?=w353:bool)
                  n193 = Equal?(x=w352, y=w346) -> (x = y?=w354:bool)
                  n194 = And(x=w354, y=w353) -> (x .and. y?=w344:bool)
                  n195 = case shown="True" w344 {
                    selector: w344 -> [_ w356]
                    tunnel: [w355 w356] -> w343
                    tunnel: w342 -> [w355 _]
                    frame False {
                    }
                    frame True {
                    }
                  }
                }
                n196 = case shown="False" w317 {
                  tunnel: w318 -> [w362 w364]
                  tunnel: [w361 w364] -> w336
                  tunnel: w328 -> [w360 _]
                  tunnel: w316 -> [w359 w363]
                  tunnel: [w358 w363] -> w315
                  frame False {
                    n197 = Build Array (concatenate)(w362, w360) -> (w361:dbl[][])
                    n198 = Build Array (concatenate)(w359, string[] ["", "", "", " ", "", "", "", " ", "", "", "", " ", "", "", "", ""] ("Valve_Status")) -> (w358:string[][])
                  }
                  frame True {
                  }
                }
                n199 = Build Array (concatenate)(w313, dbl[] [0.0, 0.0, 0.0] ("Call_List")) -> (w327:dbl[][])
                n200 = Build Array (concatenate)(w309, dbl[] [0.0, 0.0, 0.0, 0.0, 0.0, 0.0] ("Call_List")) -> (w337:dbl[][])
                n201 = Build Array (concatenate)(w311, string[] ["", "", " ", " "] ("Valve_Status")) -> (w310:string[][])
              }
              n202 = global write "DIsco_Globals.vi" "Pump_Limits"(w303) -> ()
              n203 = global write "DIsco_Globals.vi" "Pump_Data"(w299) -> ()
              n204 = global write "DIsco_Globals.vi" "Pump_Status"(w296) -> ()
              n205 = global write "DIsco_Globals.vi" "Call_List"(w305) -> ()
              n206 = global write "DIsco_Globals.vi" "Valve_Status"(w301) -> ()
            }
          }
        }
        frame #4 {
          # "Initialize Standard Variables"
          n207 = case shown="True" w365 {
            frame False {
            }
            frame True {
              n208 = flat-sequence {
                frame #0 {
                  n209 = global write "DIsco_Globals.vi" "V_Names"(string[] [] ("V_Names")) -> ()
                  n210 = global write "DIsco_Globals.vi" "V_Values"(dbl[] [] ("V_Values")) -> ()
                  n211 = global write "DIsco_Globals.vi" "V_Index"(i32[][] [] ("V_Values")) -> ()
                }
                frame #1 {
                  n212 = call "DIsco_SetVar.vi"("NewValue"=0.0, "AccessName"="Time") -> ()  [unwired: 3 in, 1 out]
                }
                frame #2 {
                  n213 = call "DIsco_VarAutoUpdate.vi"() -> ()  [unwired: 12 in]
                }
                frame #3 {
                  n214 = global read "DIsco_Globals.vi" "Pump_List"() -> (w378:string[][])
                  n215 = Array Size(array=w378) -> (size(s)=w377:i32[])
                  n216 = Index Array(array=w377, index=0) -> (element=w371:i32)
                  n217 = for {
                    N: w371 -> [_]
                    shift-right: [w382] -> w372
                    shift-left: i32[][] [[0, 0], [1, 1]] ("V_Index") -> [w383]
                    shift-right: [w385] -> _
                    shift-left: 2 ("index") -> [w386]
                    shift-right: [w380] -> w373
                    shift-left: string[] ["Time", "Date"] ("History_Headers") -> [w381]
                    n218 = for {
                      N: 3 -> [_]
                      shift-right: [w395] -> w385
                      shift-left: w386 -> [w391]
                      shift-right: [w392] -> w382
                      shift-left: w383 -> [w393]
                      shift-right: [w388] -> w380
                      shift-left: w381 -> [w389]
                      n219 = global read "DIsco_Globals.vi" "V_Names"() -> (w387:string[])
                      n220 = Build Array(w391, w391) -> (w394:i32[])
                      n221 = Increment(x=w391) -> (x+1=w395:i32)
                      n222 = Index Array(array=w387, index=w391) -> (element=w390:string)
                      n223 = Build Array (concatenate)(w389, w390) -> (w388:string[])
                      n224 = Build Array (concatenate)(w393, w394) -> (w392:i32[][])
                    }
                  }
                  n225 = global write "DIsco_Globals.vi" "History_Headers"(w373) -> ()
                  n226 = global write "DIsco_Globals.vi" "V_Index"(w372) -> ()
                }
              }
            }
          }
        }
        frame #5 {
          # "Initial Controller Calls"
          n227 = flat-sequence {
            tunnel: [w406] -> w398
            tunnel: [w404] -> w396
            tunnel: [w442] -> w401
            tunnel: [w441] -> w399
            tunnel: w398 -> [w442]
            tunnel: [w440] -> w397
            tunnel: w396 -> [w440]
            tunnel: [w445] -> w400
            tunnel: w401 -> [w446]
            tunnel: w399 -> [w444]
            tunnel: w397 -> [w443]
            frame #0 {
              # "Setup"
              n228 = global read "DIsco_Globals.vi" "Call_List"() -> (w407:dbl[][])
              n229 = Array Size(array=w407) -> (size(s)=w409:i32[])
              n230 = local read "WARN"() -> (w405:bool)
              n231 = Index Array(array=w409, index=0) -> (element=w406:i32)
              n232 = for {
                N: w406 -> [_]
                shift-right: [w410] -> w404
                shift-left: w405 -> [w411]
                i -> [w413]
                n233 = for {
                  N: 1 -> [_]
                  tunnel: w413 -> [w422]
                  shift-right: [w414] -> w410
                  shift-left: w411 -> [w415]
                  n234 = stacked-sequence {
                    tunnel: w422 -> [w424 w427 w431 w435 w438]
                    tunnel: [w423 _ _ _ _] -> w417
                    tunnel: [_ w426 _ _ _] -> w418
                    tunnel: [_ _ w430 _ _] -> w419
                    tunnel: [_ _ _ w434 _] -> w420
                    tunnel: [_ _ _ _ w437] -> w421
                    frame #0 {
                      # "Set to Remote Control"
                      n235 = call "DIsco_Comms.vi"("DIsco Command"="REMOTE", "Call Index"=w424) -> ("Checksum"=w423:bool)  [unwired: 11 in, 2 out]
                    }
                    frame #1 {
                      # "Set to Units to kPa"
                      n236 = call "DIsco_Comms.vi"("DIsco Command"="UNITS=", "Call Index"=w427, "DIsco Append"="KPA" ("DIsco_Command")) -> ("Checksum"=w426:bool)  [unwired: 10 in, 2 out]
                    }
                    frame #2 {
                      # "Set to Units to mL/min"
                      n237 = call "DIsco_Comms.vi"("DIsco Command"="UNITS=", "Call Index"=w431, "DIsco Append"="ML/MIN" ("DIsco_Command")) -> ("Checksum"=w430:bool)  [unwired: 10 in, 2 out]
                    }
                    frame #3 {
                      # "Identify Pumps"
                      n238 = call "DIsco_Comms.vi"("DIsco Command"="IDENTIFY", "Call Index"=w435) -> ("Checksum"=w434:bool)  [unwired: 11 in, 2 out]
                    }
                    frame #4 {
                      # "Get Digital Control Status"
                      n239 = call "DIsco_Comms.vi"("DIsco Command"="DIGITAL CTRL", "Call Index"=w438) -> ("Checksum"=w437:bool)  [unwired: 11 in, 2 out]
                    }
                  }
                  n240 = Compound Arithmetic op=AND(w421, w420, w419, w418, w417) -> (w416:bool)
                  n241 = Select(t=w415, s=w416, f=w416) -> (s? t:f=w414:bool)
                  "WARN" <- w414
                }
              }
            }
            frame #1 {
              n242 = Tick Count (ms)() -> (millisecond timer value=w441:u32)
            }
            frame #2 {
              # "Routine Call"
              n243 = for {
                N: w446 -> [_]
                shift-right: [w452] -> w445
                shift-left: w444 -> [w452]
                shift-right: [w447] -> _
                shift-left: w443 -> [w448]
                i -> [w453]
                n244 = stacked-sequence {
                  tunnel: w453 -> [w456 w458]
                  tunnel: [w454 _] -> w450
                  tunnel: [_ w457] -> w451
                  frame #0 {
                    # "Get All"
                    n245 = call "DIsco_Comms.vi"("DIsco Command"="GET ALL", "Call Index"=w456) -> ("Checksum"=w454:bool)  [unwired: 11 in, 2 out]
                  }
                  frame #1 {
                    # "Get Digital Status"
                    n246 = call "DIsco_Comms.vi"("DIsco Command"="DIGITAL", "Call Index"=w458) -> ("Checksum"=w457:bool)  [unwired: 11 in, 2 out]
                  }
                }
                n247 = Compound Arithmetic op=AND(w451, w450) -> (w449:bool)
                n248 = Select(t=w448, s=w449, f=w449) -> (s? t:f=w447:bool)
                n249 = local write "WARN"(w447) -> ()
              }
            }
          }
          n250 = local write "Remote Indicator"(TRUE ("Remote Indicator")) -> ()
          n251 = local write "Remote"(TRUE ("Remote")) -> ()
        }
        frame #6 {
          # "Optimize Call Rate"
          n252 = Tick Count (ms)() -> (millisecond timer value=w465:u32)
          n253 = Subtract(x=w465, y=w464) -> (x-y=w470:u32)
          n254 = Add(x=w470, y=u32 400) -> (x+y=w467:u32)
          n255 = local write "Call Execution Time (ms)"(w470) -> ()
          n256 = To Double Precision Float(number=w467) -> (double precision float=w469:dbl)
          n257 = Divide(x=w469, y=1000.0 ("x")) -> (x/y=w463:dbl)
          n258 = Round Toward +Infinity(x=w463) -> (ceil(x): smallest int >= x=w462:dbl)
          n259 = Reciprocal(x=w462) -> (1/x=w461:dbl)
          n260 = case shown="True" w460 {
            tunnel: w461 -> [w471 _]
            frame True {
              n261 = local write "Data Call Rate"(w471) -> ()
            }
            frame False {
            }
          }
        }
        frame #7 {
          # "Initial Pump Calls"
          n262 = global read "DIsco_Globals.vi" "Pump_List"() -> (w473:string[][])
          n263 = Array Size(array=w473) -> (size(s)=w476:i32[])
          n264 = local read "WARN"() -> (w472:bool)
          n265 = Index Array(array=w476, index=0) -> (element=w474:i32)
          n266 = for {
            N: w474 -> [_]
            tunnel: w473 -> [_]
            shift-right: [w482] -> _
            shift-left: w472 -> [w477]
            i -> [w483]
            n267 = stacked-sequence {
              tunnel: w483 -> [w485 w489]
              tunnel: [w484 _] -> w479
              tunnel: [_ w488] -> w480
              tunnel: [_ w487] -> w481
              frame #0 {
                # "Get Limits"
                n268 = call "DIsco_Comms.vi"("DIsco Command"="LIMITS", "Pump Index"=w485) -> ("Checksum"=w484:bool)  [unwired: 11 in, 2 out]
              }
              frame #1 {
                # "Get Setpoints"
                n269 = call "DIsco_Comms.vi"("DIsco Command"="SP", "Pump Index"=w489) -> ("Checksum"=w488:bool)  [unwired: 11 in, 2 out]
                n270 = call "DIsco_Comms.vi"("DIsco Command"="SQ", "Pump Index"=w489) -> ("Checksum"=w487:bool)  [unwired: 11 in, 2 out]
              }
            }
            n271 = Compound Arithmetic op=AND(w481, w480, w479) -> (w478:bool)
            n272 = Select(t=w477, s=w478, f=w478) -> (s? t:f=w482:bool)
          }
        }
        frame #8 {
          # "Set Controls"
          n273 = case shown="True" w492 {
            frame False {
            }
            frame True {
              n274 = global read "DIsco_Globals.vi" "Pump_List"() -> (w503:string[][])
              n275 = Array Size(array=w503) -> (size(s)=w502:i32[])
              n276 = Index Array(array=w502, index=0) -> (element=w504:i32)
              n277 = case shown="4" w504 {
                frame 0, Default {
                  w505 = ""
                  n278 = local write "Num Points 3"(100 ("Num Points 3")) -> ()
                  n279 = local write "Y1"(w505) -> ()
                  n280 = local write "Y2"(w505) -> ()
                  n281 = local write "Y3"(w505) -> ()
                  n282 = local write "Y4"(w505) -> ()
                  n283 = local write "Y5"(w505) -> ()
                  n284 = local write "Y6"(w505) -> ()
                  n285 = local write "Min Log"(0.1 ("Min Log")) -> ()
                  n286 = local write "Min_Y 3"(0.0 ("Min_Y 3")) -> ()
                  n287 = local write "Max Log"(1.0 ("Max Log")) -> ()
                  n288 = local write "Max_Y 3"(1.0 ("Max_Y 3")) -> ()
                }
                frame 1 {
                  w513 = ""
                  w515 = 0 ("index (row)")
                  n289 = local write "Num Points 3"(100 ("Num Points 3")) -> ()
                  n290 = local write "Y1"("P0" ("Y1")) -> ()
                  n291 = local write "Y2"(w513) -> ()
                  n292 = local write "Y3"(w513) -> ()
                  n293 = local write "Y4"(w513) -> ()
                  n294 = local write "Y5"("Q0" ("logY5")) -> ()
                  n295 = local write "Y6"(w513) -> ()
                  n296 = global read "DIsco_Globals.vi" "Pump_Limits"() -> (w516:dbl[][])
                  n297 = Index Array(array=w516, index (row)=w515, index (col)=1 ("disabled index (col)")) -> (element=w519:dbl)
                  n298 = Index Array(array=w516, index (row)=w515, index (col)=3 ("disabled index (col)")) -> (element=w517:dbl)
                  n299 = local write "Min Log"(1e-05 ("Min Log")) -> ()
                  n300 = local write "Min_Y 3"(0.0 ("Min_Y 3")) -> ()
                  n301 = local write "Max Log"(w517) -> ()
                  n302 = local write "Max_Y 3"(w519) -> ()
                }
                frame 2 {
                  w527 = ""
                  w529 = 0 ("index (row)")
                  n303 = local write "Num Points 3"(100 ("Num Points 3")) -> ()
                  n304 = local write "Y1"("P0" ("Y1")) -> ()
                  n305 = local write "Y2"("P1" ("logY5")) -> ()
                  n306 = local write "Y3"(w527) -> ()
                  n307 = local write "Y4"(w527) -> ()
                  n308 = local write "Y5"("Q0" ("logY5")) -> ()
                  n309 = local write "Y6"("Q1" ("logY5")) -> ()
                  n310 = global read "DIsco_Globals.vi" "Pump_Limits"() -> (w530:dbl[][])
                  n311 = Index Array(array=w530, index (row)=w529, index (col)=1 ("disabled index (col)")) -> (element=w533:dbl)
                  n312 = Index Array(array=w530, index (row)=w529, index (col)=3 ("disabled index (col)")) -> (element=w531:dbl)
                  n313 = local write "Min Log"(1e-05 ("Min Log")) -> ()
                  n314 = local write "Min_Y 3"(0.0 ("Min_Y 3")) -> ()
                  n315 = local write "Max Log"(w531) -> ()
                  n316 = local write "Max_Y 3"(w533) -> ()
                }
                frame 3 {
                  w544 = 0 ("index (row)")
                  n317 = local write "Num Points 3"(100 ("Num Points 3")) -> ()
                  n318 = local write "Y1"("P0" ("Y1")) -> ()
                  n319 = local write "Y2"("P1" ("logY5")) -> ()
                  n320 = local write "Y3"("P2" ("logY5")) -> ()
                  n321 = local write "Y4"("") -> ()
                  n322 = local write "Y5"("Q0" ("logY5")) -> ()
                  n323 = local write "Y6"("Q1" ("logY5")) -> ()
                  n324 = global read "DIsco_Globals.vi" "Pump_Limits"() -> (w545:dbl[][])
                  n325 = Index Array(array=w545, index (row)=w544, index (col)=1 ("disabled index (col)")) -> (element=w548:dbl)
                  n326 = Index Array(array=w545, index (row)=w544, index (col)=3 ("disabled index (col)")) -> (element=w546:dbl)
                  n327 = local write "Min Log"(1e-05 ("Min Log")) -> ()
                  n328 = local write "Min_Y 3"(0.0 ("Min_Y 3")) -> ()
                  n329 = local write "Max Log"(w546) -> ()
                  n330 = local write "Max_Y 3"(w548) -> ()
                }
                frame 4 {
                  w559 = 0 ("index (row)")
                  n331 = local write "Num Points 3"(100 ("Num Points 3")) -> ()
                  n332 = local write "Y1"("P0" ("Y1")) -> ()
                  n333 = local write "Y2"("P1" ("logY5")) -> ()
                  n334 = local write "Y3"("P2" ("logY5")) -> ()
                  n335 = local write "Y4"("P3" ("logY5")) -> ()
                  n336 = local write "Y5"("Q0" ("logY5")) -> ()
                  n337 = local write "Y6"("Q1" ("logY5")) -> ()
                  n338 = global read "DIsco_Globals.vi" "Pump_Limits"() -> (w560:dbl[][])
                  n339 = Index Array(array=w560, index (row)=w559, index (col)=1 ("disabled index (col)")) -> (element=w563:dbl)
                  n340 = Index Array(array=w560, index (row)=w559, index (col)=3 ("disabled index (col)")) -> (element=w561:dbl)
                  n341 = local write "Min Log"(1e-05 ("Min Log")) -> ()
                  n342 = local write "Min_Y 3"(0.0 ("Min_Y 3")) -> ()
                  n343 = local write "Max Log"(w561) -> ()
                  n344 = local write "Max_Y 3"(w563) -> ()
                }
              }
              n345 = local write "X"("Time" ("X")) -> ()
            }
          }
          n346 = global read "DIsco_Globals.vi" "Pump_List"() -> (w499:string[][])
          n347 = Array Size(array=w499) -> (size(s)=w498:i32[])
          n348 = Index Array(array=w498, index=0) -> (element=w496:i32)
          n349 = call "GetDate1900.vi"() -> ("current time (1900)"=w493:dbl)  [unwired: 1 in]
          n350 = local write "INIT"(FALSE ("INIT")) -> ()
          n351 = local write "Start Time"(w493) -> ()
          n352 = Decrement(x=w496) -> (x-1=w495:i32)
          n353 = property on="Pump Index" class="DigNum (strict)"("Maximum"=w495) -> ()  [unwired: 2 in, 2 out]
        }
        frame #9 {
          # "Import Programs"
          n354 = flat-sequence {
            frame #0 {
              n355 = call <vilib>:"Application Directory.vi"() -> ("Application Directory"=w572:path)
              n356 = Build Path(base path=w572, name or relative path="programs\\") -> (appended path=w567:path)
              n357 = List Folder(path=w567, pattern="*.csv") -> (filenames=w570:string[], error out=w569:errorcluster)  [unwired: 2 in, 2 out]
              n358 = Unbundle By Name(w569) -> ("status"=w568:bool)
              n359 = case shown="False" w568 {
                tunnel: w570 -> [w575 _]
                tunnel: w567 -> [w574 _]
                frame False {
                  n360 = for {
                    tunnel: w575 -> [w578] mode=indexing
                    tunnel: w574 -> [w579]
                    n361 = Build Path(base path=w579, name or relative path=w578) -> (appended path=w577:path)
                    n362 = Read from Text File(file (use dialog)=w577) -> (refnum out=w581:refnum<file>, text=w580:string, cancelled=w576:bool)  [unwired: 3 in, 1 out]
                    n363 = case shown="False" w576 {
                      tunnel: w580 -> [w582 _]
                      tunnel: w581 -> [w591 _]
                      frame False {
                        n364 = Refnum to Path(1:w591) -> (0:w590:path)
                        n365 = Strip Path(path=w590) -> (name=w585:string)  [unwired: 1 out]
                        n366 = Spreadsheet String To Array(delimiter (Tab)=",", format string="%g", spreadsheet string=w582, array type (2D Dbl)=string[][] []) -> (array=w583:string[][])
                        n367 = String Length(string=w585) -> (length=w589:i32)
                        n368 = Subtract(x=w589, y=4) -> (x-y=w587:i32)
                        n369 = String Subset(string=w585, offset (0)=0, length (rest)=w587) -> (substring=w584:string)
                        n370 = call "DIsco_AddProgram.vi"("Program Edit Table"=w583, "Program Name"=w584) -> ()  [unwired: 8 in, 2 out]
                      }
                      frame True {
                      }
                    }
                  }
                }
                frame True {
                  n371 = call <vilib>:"Application Directory.vi"() -> ("Application Directory"=w596:path)
                  n372 = Build Path(base path=w596, name or relative path="programs") -> (appended path=w595:path)
                  n373 = Create Folder(path (use dialog)=w595) -> ()  [unwired: 2 in, 3 out]
                  n374 = One Button Dialog(message="Warning: Pump routines database not found.", button name ("OK")="OK") -> ()  [unwired: 1 out]
                }
              }
            }
            frame #1 {
              # "Set Maximum Range"
              n375 = global read "DIsco_Globals.vi" "Program Names"() -> (w602:string[])
              n376 = Array Size(array=w602) -> (size(s)=w601:i32)
              n377 = Decrement(x=w601) -> (x-1=w600:i32)
              n378 = property on="Program Selector" class="DigNum (strict)"("Maximum"=w600) -> ()  [unwired: 2 in, 2 out]
            }
          }
        }
        frame #10 {
          # "Pump Matrix Headers"
          n379 = global read "DIsco_Globals.vi" "Pump_List"() -> (w605:string[][])
          n380 = for {
            tunnel: w605 -> [_] mode=indexing
            shift-right: [w607] -> w603
            shift-left: string[] [] ("Row Header Strings[]") -> [w606]
            i -> [w609]
            n381 = Number To Decimal String(number=w609) -> (decimal integer string=w608:string)  [unwired: 1 in]
            n382 = Build Array (concatenate)(w606, w608) -> (w607:string[])
          }
          n383 = property on="Pump Matrix" class="Tbl (strict)"("Row Headers[]"=w603) -> ()  [unwired: 2 in, 2 out]
        }
        frame #11 {
          # "Warning popup"
          n384 = local read "WARN"() -> (w610:bool)
          n385 = case shown="False" w610 {
            frame False {
              n386 = Two Button Dialog(message="!!! Warning !!! Communication failure during startup", 1:"Continue anyway" ("F button name (\"Cancel\")"), 2:"Exit now" ("T button name (\"OK\")")) -> (T button?=w612:bool)
              n387 = local write "WARN"(TRUE ("WARN")) -> ()
              n388 = local write "stop"(w612) -> ()
            }
            frame True {
            }
          }
        }
      }
    }
    frame #1 {
      # "User Interface Thread"
      # "Pump Command Thread"
      n389 = while {
        stop <- w620 stop-if-true
        n390 = stacked-sequence {
          frame #0 {
            # "Rename Pump"
            n391 = case shown="True" "RenamePump" {
              frame False {
              }
              frame True {
                n392 = local read "Pump Index"() -> (w624:i32)
                n393 = global read "DIsco_Globals.vi" "Pump_List"() -> (w628:string[][])
                n394 = Replace Array Subset(array=w628, new element="Rename", index (row)=w624, index (col)=0 ("disabled index (col)")) -> (w627:string[][])
                n395 = global write "DIsco_Globals.vi" "Pump_List"(w627) -> ()
                n396 = property on="RenamePump" class="Bool (strict)"("Value"=FALSE ("RenamePump")) -> ()  [unwired: 2 in, 2 out]
              }
            }
          }
          frame #1 {
            # "Reset History Data"
            n397 = case shown="True" "HistData Clear" {
              frame False {
              }
              frame True {
                n398 = global read "DIsco_Globals.vi" "Pump_List"() -> (w650:string[][])
                n399 = global read "DIsco_Globals.vi" "V_Names"() -> (w637:string[])
                n400 = global read "DIsco_Globals.vi" "Call_List"() -> (w645:dbl[][])
                n401 = global read "DIsco_Globals.vi" "V_Values"() -> (w632:dbl[])
                n402 = call "GetDate1900.vi"() -> ("current time (1900)"=w630:dbl)  [unwired: 1 in]
                n403 = Array Size(array=w650) -> (size(s)=w649:i32[])
                n404 = Array Size(array=w645) -> (size(s)=w646:i32[])
                n405 = global write "DIsco_Globals.vi" "History_Headers"(string[] ["Time", "Date"] ("History_Headers")) -> ()
                n406 = global write "DIsco_Globals.vi" "History_Data"(dbl[][] [] ("History_Data")) -> ()
                n407 = global write "DIsco_Globals.vi" "V_Index"(i32[][] [[0, 0], [1, 1]] ("V_Index")) -> ()
                n408 = global write "DIsco_Globals.vi" "E_Names"(string[] [] ("E_Names")) -> ()
                n409 = global write "DIsco_Globals.vi" "E_Cols"(i32[] [] ("E_Cols")) -> ()
                n410 = global write "DIsco_Globals.vi" "E_Index"(i32[][] [] ("V_Index")) -> ()
                n411 = global write "DIsco_Globals.vi" "E_Paths"(path[] [] ("E_Paths")) -> ()
                n412 = global write "DIsco_Globals.vi" "E_Vals"(dbl[] [] ("E_Vals")) -> ()
                n413 = local write "Start Time"(w630) -> ()
                n414 = Index Array(array=w649, index=0) -> (element=w644:i32)
                n415 = Index Array(array=w646, index=0) -> (element=w639:i32)
                n416 = Multiply(x=w644, y=11) -> (x*y=w641:i32)
                n417 = Multiply(x=w639, y=8) -> (x*y=w638:i32)
                n418 = property on="HistData Clear" class="Bool (strict)"("Value"=FALSE ("HistData Clear")) -> ()  [unwired: 2 in, 2 out]
                n419 = Compound Arithmetic op=ADD(2 ("index"), w641, w638) -> (w631:i32)
                n420 = Array Subset(array=w637, index=0, length=w631) -> (w635:string[])
                n421 = Array Subset(array=w632, index=0, length=w631) -> (w634:dbl[])
                n422 = global write "DIsco_Globals.vi" "V_Names"(w635) -> ()
                n423 = global write "DIsco_Globals.vi" "V_Values"(w634) -> ()
              }
            }
          }
          frame #2 {
            # "Empty History Data"
            n424 = case shown="True" "HistData Empty" {
              frame False {
              }
              frame True {
                n425 = call "GetDate1900.vi"() -> ("current time (1900)"=w661:dbl)  [unwired: 1 in]
                n426 = global write "DIsco_Globals.vi" "History_Data"(dbl[][] [] ("History_Data")) -> ()
                n427 = property on="HistData Empty" class="Bool (strict)"("Value"=FALSE ("HistData Clear")) -> ()  [unwired: 2 in, 2 out]
                n428 = local write "Start Time"(w661) -> ()
              }
            }
          }
          frame #3 {
            # "Clear External Data"
            n429 = case shown="True" "ExtData Clear" {
              frame False {
              }
              frame True {
                n430 = global write "DIsco_Globals.vi" "E_Names"(string[] [] ("E_Names")) -> ()
                n431 = global write "DIsco_Globals.vi" "E_Cols"(i32[] [] ("E_Cols")) -> ()
                n432 = global write "DIsco_Globals.vi" "E_Paths"(path[] [] ("E_Paths")) -> ()
                n433 = global write "DIsco_Globals.vi" "E_Vals"(dbl[] [] ("E_Vals")) -> ()
                n434 = global write "DIsco_Globals.vi" "E_Index"(i32[][] [] ("E_Cols")) -> ()
                n435 = property on="ExtData Clear" class="Bool (strict)"("Value"=FALSE ("HistData Clear")) -> ()  [unwired: 2 in, 2 out]
              }
            }
          }
          frame #4 {
            # "Fetch pump information with selector change"
            n436 = local read "Pump Index"() -> (w671:i32)
            n437 = local read "Fetch"() -> (w673:i32)
            n438 = Not Equal?(x=w673, y=w671) -> (x != y?=w672:bool)
            n439 = case shown="True" w672 {
              tunnel: w671 -> [_ w674]
              frame False {
              }
              frame True {
                n440 = stacked-sequence {
                  tunnel: w674 -> [w678 w754]
                  frame #0 {
                    n441 = global read "DIsco_Globals.vi" "Pump_Status"() -> (w683:string[][])
                    n442 = local write "Fetch"(w678) -> ()
                    n443 = Number To Decimal String(number=w678) -> (decimal integer string=w702:string)  [unwired: 1 in]
                    n444 = Number To Decimal String(number=w678) -> (decimal integer string=w705:string)  [unwired: 1 in]
                    n445 = global read "DIsco_Globals.vi" "Pump_Limits"() -> (w695:dbl[][])
                    n446 = Index Array(array=w683, index (row)=w678, index (col)=3 ("disabled index (col)")) -> (element=w682:string)
                    n447 = global read "DIsco_Globals.vi" "Pump_Data"() -> (w689:dbl[][])
                    n448 = global read "DIsco_Globals.vi" "Pump_Data"() -> (w691:dbl[][])
                    n449 = global read "DIsco_Globals.vi" "Pump_Data"() -> (w693:dbl[][])
                    n450 = case shown="\"CP\"" w682 {
                      frame "CP" {
                        n451 = local write "CCF Ind"(FALSE ("CCF Ind")) -> ()
                        n452 = local write "CCP Ind"(FALSE ("CCF Ind")) -> ()
                        n453 = local write "CF Ind"(FALSE ("CCF Ind")) -> ()
                        n454 = local write "CP Ind"(TRUE ("CCP Ind")) -> ()
                        n455 = local write "CF"(FALSE ("Constant Flow")) -> ()
                        n456 = local write "CP"(TRUE ("CCP Ind")) -> ()
                        n457 = local write "CCF"(FALSE ("CCP")) -> ()
                        n458 = local write "CCP"(FALSE ("Constant Pressure")) -> ()
                      }
                      frame "UNK", Default {
                        n459 = local write "CCF Ind"(FALSE ("CCF Ind")) -> ()
                        n460 = local write "CCP Ind"(FALSE ("CCF Ind")) -> ()
                        n461 = local write "CF Ind"(FALSE ("CCF Ind")) -> ()
                        n462 = local write "CP Ind"(FALSE ("CCP Ind")) -> ()
                        n463 = local write "CF"(FALSE ("Constant Flow")) -> ()
                        n464 = local write "CP"(FALSE ("CCP Ind")) -> ()
                        n465 = local write "CCF"(FALSE ("CCP")) -> ()
                        n466 = local write "CCP"(FALSE ("Constant Pressure")) -> ()
                      }
                      frame "CF" {
                        n467 = local write "CCF Ind"(FALSE ("CCF Ind")) -> ()
                        n468 = local write "CCP Ind"(FALSE ("CCF Ind")) -> ()
                        n469 = local write "CF Ind"(TRUE ("CCF Ind")) -> ()
                        n470 = local write "CP Ind"(FALSE ("CCP Ind")) -> ()
                        n471 = local write "CF"(TRUE ("Constant Flow")) -> ()
                        n472 = local write "CP"(FALSE ("CCP Ind")) -> ()
                        n473 = local write "CCF"(FALSE ("CCP")) -> ()
                        n474 = local write "CCP"(FALSE ("Constant Pressure")) -> ()
                      }
                      frame "CCP" {
                        n475 = local write "CCF Ind"(FALSE ("CCF Ind")) -> ()
                        n476 = local write "CCP Ind"(TRUE ("CCF Ind")) -> ()
                        n477 = local write "CF Ind"(FALSE ("CCF Ind")) -> ()
                        n478 = local write "CP Ind"(FALSE ("CCP Ind")) -> ()
                        n479 = local write "CF"(FALSE ("Constant Flow")) -> ()
                        n480 = local write "CP"(FALSE ("CCP Ind")) -> ()
                        n481 = local write "CCF"(FALSE ("CCP")) -> ()
                        n482 = local write "CCP"(TRUE ("Constant Pressure")) -> ()
                      }
                      frame "CCF" {
                        n483 = local write "CCF Ind"(TRUE ("CCF Ind")) -> ()
                        n484 = local write "CCP Ind"(FALSE ("CCF Ind")) -> ()
                        n485 = local write "CF Ind"(FALSE ("CCF Ind")) -> ()
                        n486 = local write "CP Ind"(FALSE ("CCP Ind")) -> ()
                        n487 = local write "CF"(FALSE ("Constant Flow")) -> ()
                        n488 = local write "CP"(FALSE ("CCP Ind")) -> ()
                        n489 = local write "CCF"(TRUE ("CCP")) -> ()
                        n490 = local write "CCP"(FALSE ("Constant Pressure")) -> ()
                      }
                    }
                    n491 = Concatenate Strings("SQ", w702) -> (w704:string)
                    n492 = Concatenate Strings("SP", w705) -> (w707:string)
                    n493 = call "DIsco_GetCustomVar.vi"("Name"=w704) -> ("ValueFound"=w681:dbl)  [unwired: 2 in, 2 out]
                    n494 = call "DIsco_GetCustomVar.vi"("Name"=w707) -> ("ValueFound"=w680:dbl)  [unwired: 2 in, 2 out]
                    n495 = Index Array(array=w683, index (row)=w678) -> (element=w675:string[])  [unwired: 1 in]
                    n496 = Index Array(array=w675, index=1) -> (element=w676:string)
                    n497 = case shown="\"L\", Default" w676 {
                      frame "L", Default {
                        w708 = FALSE ("Remote")
                        n498 = local write "Remote Indicator"(w708) -> ()
                        n499 = local write "Remote"(w708) -> ()
                      }
                      frame "R" {
                        w709 = TRUE ("Remote")
                        n500 = local write "Remote Indicator"(w709) -> ()
                        n501 = local write "Remote"(w709) -> ()
                      }
                    }
                    n502 = Index Array(array=w689, index (row)=w678, index (col)=0 ("disabled index (col)")) -> (element=w688:dbl)
                    n503 = Index Array(array=w691, index (row)=w678, index (col)=1 ("disabled index (col)")) -> (element=w687:dbl)
                    n504 = Index Array(array=w693, index (row)=w678, index (col)=2 ("disabled index (col)")) -> (element=w686:dbl)
                    n505 = Index Array(array=w695, index (row)=w678, index (col)=5 ("disabled index (col)")) -> (element=w697:dbl)
                    n506 = local write "Flow Setpoint"(w681) -> ()
                    n507 = local write "Pressure Setpoint"(w680) -> ()
                    n508 = call "Parse_Status.vi"("Abbr Status"=w675) -> ("Full Status"=w679:string[])  [unwired: 10 in]
                    n509 = local write "P Active"(w688) -> ()
                    n510 = local write "F Active"(w687) -> ()
                    n511 = local write "V Active"(w686) -> ()
                    n512 = Divide(x=w686, y=w697) -> (x/y=w701:dbl)
                    n513 = Multiply(x=w701, y=100.0) -> (x*y=w699:dbl)
                    n514 = Subtract(x=100.0, y=w699) -> (x-y=w685:dbl)
                    n515 = local write "Status"(w679) -> ()
                    n516 = local write "Vol %"(w685) -> ()
                  }
                  frame #1 {
                    n517 = call "DIsco_PumpListParse.vi"("Pump Index In"=w754) -> ("Pump Type"=w758:string, "Call Index"=w750:i32, "Pump Name"=w757:string, "Pump Letter"=w756:string)  [unwired: 6 in, 5 out]
                    n518 = global read "DIsco_Globals.vi" "Pump_Status"() -> (w755:string[][])
                    n519 = local write "Name of Selected Pump"(w757) -> ()
                    n520 = local write "Pump Type"(w758) -> ()
                    n521 = local write "Call ID"(w750) -> ()
                    n522 = local write "Rename"(w757) -> ()
                    n523 = local write "Letter"(w756) -> ()
                    n524 = Index Array(array=w755, index (row)=w754, index (col)=3 ("disabled index (col)")) -> (element=w752:string)
                    n525 = case shown="\"A\", Default" w756 {
                      tunnel: w752 -> [w760 _]
                      frame "B" {
                        n526 = case shown="\"CCF\"" w760 {
                          frame "CF", Default {
                            w761 = T2."Enabled" ("Disabled")
                            w762 = T2."Disabled and Grayed Out" ("Disabled")
                            n527 = property on="CCF" class="Bool (strict)"("DisabledEnum"=w762) -> ()  [unwired: 2 in, 2 out]
                            n528 = property on="CCP" class="Bool (strict)"("DisabledEnum"=w762) -> ()  [unwired: 2 in, 2 out]
                            n529 = property on="CP" class="Bool (strict)"("DisabledEnum"=w761) -> ()  [unwired: 2 in, 2 out]
                            n530 = property on="CF" class="Bool (strict)"("DisabledEnum"=w761) -> ()  [unwired: 2 in, 2 out]
                          }
                          frame "CP" {
                            w763 = T2."Enabled" ("Disabled")
                            w764 = T2."Disabled and Grayed Out" ("Disabled")
                            n531 = property on="CCF" class="Bool (strict)"("DisabledEnum"=w764) -> ()  [unwired: 2 in, 2 out]
                            n532 = property on="CCP" class="Bool (strict)"("DisabledEnum"=w764) -> ()  [unwired: 2 in, 2 out]
                            n533 = property on="CP" class="Bool (strict)"("DisabledEnum"=w763) -> ()  [unwired: 2 in, 2 out]
                            n534 = property on="CF" class="Bool (strict)"("DisabledEnum"=w763) -> ()  [unwired: 2 in, 2 out]
                          }
                          frame "CCF" {
                            w765 = T2."Disabled and Grayed Out" ("Disabled")
                            n535 = property on="CCF" class="Bool (strict)"("DisabledEnum"=w765) -> ()  [unwired: 2 in, 2 out]
                            n536 = property on="CCP" class="Bool (strict)"("DisabledEnum"=w765) -> ()  [unwired: 2 in, 2 out]
                            n537 = property on="CP" class="Bool (strict)"("DisabledEnum"=w765) -> ()  [unwired: 2 in, 2 out]
                            n538 = property on="CF" class="Bool (strict)"("DisabledEnum"=w765) -> ()  [unwired: 2 in, 2 out]
                          }
                          frame "CCP" {
                            w766 = T2."Disabled and Grayed Out" ("Disabled")
                            n539 = property on="CCF" class="Bool (strict)"("DisabledEnum"=w766) -> ()  [unwired: 2 in, 2 out]
                            n540 = property on="CCP" class="Bool (strict)"("DisabledEnum"=w766) -> ()  [unwired: 2 in, 2 out]
                            n541 = property on="CP" class="Bool (strict)"("DisabledEnum"=w766) -> ()  [unwired: 2 in, 2 out]
                            n542 = property on="CF" class="Bool (strict)"("DisabledEnum"=w766) -> ()  [unwired: 2 in, 2 out]
                          }
                        }
                      }
                      frame "A", Default {
                        w767 = T2."Enabled" ("Disabled")
                        n543 = property on="CCF" class="Bool (strict)"("DisabledEnum"=w767) -> ()  [unwired: 2 in, 2 out]
                        n544 = property on="CCP" class="Bool (strict)"("DisabledEnum"=w767) -> ()  [unwired: 2 in, 2 out]
                        n545 = property on="CP" class="Bool (strict)"("DisabledEnum"=w767) -> ()  [unwired: 2 in, 2 out]
                        n546 = property on="CF" class="Bool (strict)"("DisabledEnum"=w767) -> ()  [unwired: 2 in, 2 out]
                      }
                    }
                    n547 = case shown="True" "Track Pump Index" {
                      tunnel: w750 -> [_ w759]
                      frame False {
                      }
                      frame True {
                        n548 = local write "Control ID"(w759) -> ()
                      }
                    }
                  }
                }
              }
            }
          }
          frame #5 {
            # "Browse Manual Pump Commands"
            n549 = local read "Brow"() -> (w769:i32)
            n550 = Not Equal?(x="Browse", y=w769) -> (x != y?=w768:bool)
            n551 = case shown="True" w768 {
              tunnel: "Browse" -> [_ w771]
              frame False {
              }
              frame True {
                n552 = global read "DIsco_Globals.vi" "Comms_List"() -> (w777:string[][])
                n553 = local write "Brow"(w771) -> ()
                n554 = Index Array(array=w777, index (row)=w771) -> (element=w774:string[])  [unwired: 1 in]
                n555 = Index Array(array=w774, index=0) -> (element=w772:string)
                n556 = Index Array(array=w774, index=1) -> (element=→"Description":string)
                n557 = local write "Command"(w772) -> ()
              }
            }
          }
          frame #6 {
            # "Find Manual Pump Commands"
            n558 = local read "Browse"() -> (w780:i32)
            n559 = call "DIsco_CommList.vi"("Command In"="Command") -> ("Exists?"=w783:bool, "Command Out"=w782:string, "Command Description"=w781:string, "Index"=w778:i32)  [unwired: 11 in]
            n560 = Not Equal?(x=w778, y=w780) -> (x != y?=w779:bool)
            n561 = case shown="True" w779 {
              tunnel: w783 -> [_ w788]
              tunnel: w782 -> [_ w787]
              tunnel: w781 -> [_ w786]
              tunnel: w778 -> [_ w785]
              frame False {
              }
              frame True {
                n562 = local write "Browse"(w785) -> ()
                n563 = local write "Brow"(w785) -> ()
                n564 = case shown="True" w788 {
                  tunnel: w787 -> [w789 _]
                  tunnel: w786 -> [w791 _]
                  frame True {
                    n565 = Concatenate Strings(w789, " : " ("string"), w791) -> (w790:string)
                    n566 = local write "Description"(w790) -> ()
                  }
                  frame False {
                    n567 = local write "Description"("***INVALID COMMAND***" ("Meaning")) -> ()
                  }
                }
              }
            }
          }
          frame #7 {
            # "Index Variables"
            n568 = global read "DIsco_Globals.vi" "V_Names"() -> (w795:string[])
            n569 = global read "DIsco_Globals.vi" "V_Values"() -> (w794:dbl[])
            n570 = Index Array(array=w795, index="Add V Index") -> (element=→"Var N":string)
            n571 = Index Array(array=w794, index="Add V Index") -> (element=→"Var V":dbl)
          }
          frame #8 {
            # "Add External Data to Links"
            n572 = case shown="True" "E_Add" {
              frame False {
              }
              frame True {
                n573 = local read "External File Path"() -> (w816:path)
                n574 = global read "DIsco_Globals.vi" "History_Headers"() -> (w800:string[])
                n575 = local read "External Data"() -> (w813:dbl[][])
                n576 = global read "DIsco_Globals.vi" "E_Names"() -> (w821:string[])
                n577 = global read "DIsco_Globals.vi" "E_Paths"() -> (w819:path[])
                n578 = global read "DIsco_Globals.vi" "E_Cols"() -> (w803:i32[])
                n579 = global read "DIsco_Globals.vi" "E_Vals"() -> (w815:dbl[])
                n580 = global read "DIsco_Globals.vi" "E_Index"() -> (w807:i32[][])
                n581 = Array Size(array=w803) -> (size(s)=w802:i32)
                n582 = Array Size(array=w800) -> (size(s)=w801:i32)
                n583 = Index Array(array=w813, index (row)=0, index (col)="E_Col_Index") -> (element=w809:dbl)
                n584 = Build Array (concatenate)(w821, "E_Col_Name") -> (w820:string[])
                n585 = Build Array (concatenate)(w815, w809) -> (w814:dbl[])
                n586 = Build Array (concatenate)(w800, "E_Col_Name") -> (w811:string[])
                n587 = Build Array (concatenate)(w819, w816) -> (w818:path[])
                n588 = Build Array (concatenate)(w803, "E_Col_Index") -> (w817:i32[])
                n589 = Build Array(w802, w801) -> (w805:i32[])
                n590 = Build Array (concatenate)(w807, w805) -> (w806:i32[][])
                n591 = global write "DIsco_Globals.vi" "History_Headers"(w811) -> ()
                n592 = global write "DIsco_Globals.vi" "E_Names"(w820) -> ()
                n593 = global write "DIsco_Globals.vi" "E_Paths"(w818) -> ()
                n594 = global write "DIsco_Globals.vi" "E_Cols"(w817) -> ()
                n595 = global write "DIsco_Globals.vi" "E_Vals"(w814) -> ()
                n596 = global write "DIsco_Globals.vi" "E_Index"(w806) -> ()
                n597 = property on="E_Add" class="Bool (strict)"("Value"=FALSE ("E_Add")) -> ()  [unwired: 2 in, 2 out]
              }
            }
          }
          frame #9 {
            # "Add Variable Data to History Tracker"
            n598 = case shown="True" "Add Var" {
              frame False {
              }
              frame True {
                n599 = global read "DIsco_Globals.vi" "History_Headers"() -> (w826:string[])
                n600 = local read "Add V Index"() -> (w828:i32)
                n601 = local read "Var N"() -> (w829:string)
                n602 = global read "DIsco_Globals.vi" "V_Index"() -> (w824:i32[][])
                n603 = Build Array (concatenate)(w826, w829) -> (w830:string[])
                n604 = Array Size(array=w826) -> (size(s)=w825:i32)
                n605 = Build Array(w828, w825) -> (w827:i32[])
                n606 = Build Array (concatenate)(w824, w827) -> (w823:i32[][])
                n607 = global write "DIsco_Globals.vi" "History_Headers"(w830) -> ()
                n608 = global write "DIsco_Globals.vi" "V_Index"(w823) -> ()
                n609 = property on="Add Var" class="Bool (strict)"("Value"=FALSE ("E_Add")) -> ()  [unwired: 2 in, 2 out]
              }
            }
          }
          frame #10 {
            # "Indicate Active Data Links"
            n610 = global read "DIsco_Globals.vi" "E_Index"() -> (w836:i32[][])
            n611 = Array Size(array=w836) -> (size(s)=w835:i32[])
            n612 = Index Array(array=w835, index=0) -> (element=w833:i32)
            n613 = Greater Than 0?(x=w833) -> (x > 0?=w832:bool)
            "LNK" <- w832
            n614 = property on="LNK" class="Bool (strict)"("Blinking"=w832) -> ()  [unwired: 2 in, 2 out]
          }
          frame #11 {
            # "Reset Program"
            n615 = case shown="True" "Reset" {
              frame False {
              }
              frame True {
                n616 = property on="Reset" class="Bool (strict)"("Blinking"=FALSE) -> ()  [unwired: 2 in, 2 out]
                n617 = local write "Reset"(FALSE ("Reset")) -> ()
                n618 = property on="Run Program" class="Bool (strict)"("Value"=FALSE ("Run Program")) -> ()  [unwired: 2 in, 2 out]
                n619 = local write "ERR"(TRUE ("ERR")) -> ()
                n620 = local write "Step"(0 ("Step")) -> ()
              }
            }
          }
          frame #12 {
            # "Valve/Digital Graphics"
            n621 = global read "DIsco_Globals.vi" "Valve_Status"() -> (w891:string[][])
            n622 = local read "Control ID"() -> (w876:i32)
            n623 = Index Array(array=w891, index (row)=w876) -> (element=w843:string[])  [unwired: 1 in]
            n624 = Index Array(array=w843, index=8) -> (element=w851:string)
            n625 = Index Array(array=w843, index=9) -> (element=w850:string)
            n626 = Index Array(array=w843, index=10) -> (element=w849:string)
            n627 = Index Array(array=w843, index=11) -> (element=w848:string)
            n628 = Index Array(array=w843, index=12) -> (element=w847:string)
            n629 = Index Array(array=w843, index=13) -> (element=w846:string)
            n630 = Index Array(array=w843, index=14) -> (element=w845:string)
            n631 = Index Array(array=w843, index=15) -> (element=w844:string)
            n632 = Index Array(array=w843, index=0) -> (element=w902:string)
            n633 = Index Array(array=w843, index=1) -> (element=w903:string)
            n634 = Index Array(array=w843, index=2) -> (element=w904:string)
            n635 = Index Array(array=w843, index=3) -> (element=w905:string)
            n636 = Index Array(array=w843, index=4) -> (element=w906:string)
            n637 = Index Array(array=w843, index=5) -> (element=w907:string)
            n638 = Index Array(array=w843, index=6) -> (element=w908:string)
            n639 = Index Array(array=w843, index=7) -> (element=w909:string)
            n640 = Equal?(x="I", y=w851) -> (x = y?=→"VI 16":bool)
            n641 = Equal?(x="I", y=w850) -> (x = y?=→"VI 15":bool)
            n642 = Equal?(x="I", y=w849) -> (x = y?=→"VI 14":bool)
            n643 = Equal?(x="I", y=w848) -> (x = y?=→"VI 13":bool)
            n644 = Equal?(x="I", y=w847) -> (x = y?=→"VI 12":bool)
            n645 = Equal?(x="I", y=w846) -> (x = y?=→"VI 11":bool)
            n646 = Equal?(x="I", y=w845) -> (x = y?=→"VI 10":bool)
            n647 = Equal?(x="I", y=w844) -> (x = y?=→"VI 9":bool)
            n648 = Equal?(x="H", y=w902) -> (x = y?=→"VI 1":bool)
            n649 = Equal?(x="H", y=w903) -> (x = y?=→"VI 2":bool)
            n650 = Equal?(x="H", y=w904) -> (x = y?=→"VI 3":bool)
            n651 = Equal?(x="H", y=w905) -> (x = y?=→"VI 4":bool)
            n652 = Equal?(x="H", y=w906) -> (x = y?=→"VI 5":bool)
            n653 = Equal?(x="H", y=w907) -> (x = y?=→"VI 6":bool)
            n654 = Equal?(x="H", y=w908) -> (x = y?=→"VI 7":bool)
            n655 = Equal?(x="H", y=w909) -> (x = y?=→"VI 8":bool)
          }
          frame #13 {
            # "Set Manual Variable"
            n656 = case shown="True" "Set Var" {
              frame False {
              }
              frame True {
                n657 = property on="Set Var" class="Bool (strict)"("Value"=FALSE ("Set Var")) -> ()  [unwired: 2 in, 2 out]
                n658 = call "DIsco_VariableMath.vi"("PASS VALUE"="Input Variable (Name=Function)") -> ()  [unwired: 4 in, 1 out]
              }
            }
          }
          frame #14 {
            # "Log Commands"
            n659 = global write "DIsco_Globals.vi" "Logging"("Log Commands") -> ()
          }
          frame #15 {
            # "Import Array from *.CSV File"
            n660 = case shown="True" "Import CSV" {
              frame False {
              }
              frame True {
                n661 = Read from Text File() -> (refnum out=w915:refnum<file>, text=w920:string, cancelled=w919:bool)  [unwired: 4 in, 1 out]
                n662 = Not(x=w919) -> (.not. x?=w918:bool)
                n663 = case shown="True" w918 {
                  tunnel: w920 -> [_ w930]
                  tunnel: w915 -> [_ w928]
                  frame False {
                  }
                  frame True {
                    n664 = Refnum to Path(1:w928) -> (0:w927:path)
                    n665 = Strip Path(path=w927) -> (name=w922:string)  [unwired: 1 out]
                    n666 = Spreadsheet String To Array(delimiter (Tab)=",", format string="%g", spreadsheet string=w930, array type (2D Dbl)=string[][] []) -> (array=w929:string[][])
                    n667 = String Length(string=w922) -> (length=w926:i32)
                    n668 = local write "Program Edit Table"(w929) -> ()
                    n669 = Subtract(x=w926, y=4) -> (x-y=w924:i32)
                    n670 = String Subset(string=w922, offset (0)=0, length (rest)=w924) -> (substring=w921:string)
                    n671 = local write "Routine Name"(w921) -> ()
                  }
                }
                n672 = local write "Import CSV"(FALSE ("Import CSV")) -> ()
                n673 = local write "AddIt"(TRUE ("AddIt")) -> ()
              }
            }
          }
          frame #16 {
            # "Export Selected Program as CSV"
            n674 = local read "Program Edit Table"() -> (w934:string[][])
            n675 = call "DIsco_ParseProgram.vi"("Program Array"=w934) -> ("Truncated Array"=w935:string[][])  [unwired: 8 in, 2 out]
            n676 = case shown="True" "Export" {
              tunnel: w935 -> [_ w947]
              tunnel: [errorcluster {"status"=FALSE, "code"=0, "source"=""} ("error out") w938] -> _
              frame False {
              }
              frame True {
                w943 = "*.csv" ("pattern (all files)")
                n677 = Array To Spreadsheet String(delimiter (Tab)=",", array=w947, 3:"%g" ("format string")) -> (spreadsheet string=w940:string)
                n678 = local read "Routine Name"() -> (w946:string)
                n679 = call "File Dialog"("prompt"="Save pump routine", "button label"="Save", "default name"=w946, "pattern (all files)"=w943, "pattern label"=w943) -> ("selected path"=w942:path, "cancelled"=w941:bool, "error out"=w939:errorcluster)  [unwired: 7 in, 1 out]
                n680 = case shown="False" w941 {
                  tunnel: w942 -> [w954 _]
                  tunnel: w940 -> [w953 _]
                  tunnel: w939 -> [w952 w955]
                  tunnel: [w951 w955] -> w938
                  frame False {
                    n681 = Write to Text File(file (use dialog)=w954, text=w953, error in=w952) -> (error out=w951:errorcluster)  [unwired: 1 in, 2 out]
                  }
                  frame True {
                  }
                }
                n682 = local write "Export"(FALSE ("Export")) -> ()
              }
            }
          }
          frame #17 {
            # "Add Edited Program to Database"
            n683 = case shown="True" "AddIt" {
              frame False {
              }
              frame True {
                n684 = local read "Program Selector"() -> (w957:i32)
                n685 = call "DIsco_AddProgram.vi"("Program Edit Table"="Program Edit Table", "Program Name"="Routine Name", "Selector in"=w957) -> ("Selector out"=w961:i32)  [unwired: 7 in, 1 out]
                n686 = local write "AddIt"(FALSE ("AddIt")) -> ()
                n687 = local write "Program Selector"(w961) -> ()
              }
            }
          }
          frame #18 {
            # "Program Selector"
            n688 = local read "Prog Fetch"() -> (w963:i32)
            n689 = Not Equal?(x="Program Selector", y=w963) -> (x != y?=w962:bool)
            n690 = case shown="True" w962 {
              tunnel: "Program Selector" -> [_ w968]
              frame False {
              }
              frame True {
                # "Set Maximum Range"
                n691 = global read "DIsco_Globals.vi" "Program Names"() -> (w973:string[])
                n692 = global read "DIsco_Globals.vi" "Program Stack"() -> (w969:string[][][])
                n693 = global read "DIsco_Globals.vi" "Program Names"() -> (w972:string[])
                n694 = Array Size(array=w972) -> (size(s)=w971:i32)
                n695 = Index Array(array=w973, index=w968) -> (element=w965:string)
                n696 = Index Array(array=w969, index (dim 0)=w968) -> (element=w967:string[][])  [unwired: 2 in]
                n697 = local write "Prog Fetch"(w968) -> ()
                n698 = Decrement(x=w971) -> (x-1=w970:i32)
                n699 = local write "Routine Name"(w965) -> ()
                n700 = call "DIsco_ParseProgram.vi"("Program Array"=w967) -> ("Truncated Array"=w966:string[][])  [unwired: 8 in, 2 out]
                n701 = local write "Program Edit Table"(w966) -> ()
                n702 = property on="Program Selector" class="DigNum (strict)"("Maximum"=w970) -> ()  [unwired: 2 in, 2 out]
              }
            }
          }
          frame #19 {
            # "Remove Program"
            n703 = case shown="True" "Remove" {
              frame False {
              }
              frame True {
                n704 = local write "Remove"(FALSE ("Remove")) -> ()
                n705 = Two Button Dialog(message="Are you sure?", 2:"Remove" ("T button name (\"OK\")")) -> (T button?=w976:bool)  [unwired: 1 in]
                n706 = case shown="True" w976 {
                  frame False {
                  }
                  frame True {
                    n707 = global read "DIsco_Globals.vi" "Program Names"() -> (w983:string[])
                    n708 = global read "DIsco_Globals.vi" "Program Stack"() -> (w984:string[][][])
                    n709 = local read "Program Selector"() -> (w980:i32)
                    n710 = Decrement(x=w980) -> (x-1=w979:i32)
                    n711 = Delete From Array(array=w983, index=w980) -> (array with subset deleted=w981:string[])  [unwired: 1 in, 1 out]
                    n712 = Delete From Array(array=w984, index (dim 0)=w980) -> (array with subset deleted=w982:string[][][])  [unwired: 3 in, 1 out]
                    n713 = global write "DIsco_Globals.vi" "Program Names"(w981) -> ()
                    n714 = global write "DIsco_Globals.vi" "Program Stack"(w982) -> ()
                    n715 = local write "Program Selector"(w979) -> ()
                  }
                }
              }
            }
          }
          frame #20 {
            # "Table UI Referencing"
            n716 = local read "Program Edit Table"() -> (w989:string[][])
            n717 = local read "Prev Select"() -> (w992:i32)
            n718 = property on="Program Edit Table" class="Tbl (strict)"() -> ("Selection Start"=w995:T3)  [unwired: 2 in, 2 out]
            n719 = Unbundle By Name(w995) -> ("Row"=w986:i32)
            n720 = Array Size(array=w989) -> (size(s)=w990:i32[])
            n721 = Index Array(array=w989, index (row)=w986, index (col)=0 ("disabled index (col)")) -> (element=w985:string)
            n722 = Index Array(array=w990, index=0) -> (element=w988:i32)
            n723 = Not Equal?(x=w986, y=w992) -> (x != y?=w993:bool)
            n724 = case shown="True" w993 {
              tunnel: w992 -> [_ w1004]
              tunnel: w988 -> [_ w1003]
              tunnel: string[] [] -> [_ w1002]
              tunnel: w986 -> [_ w1001]
              tunnel: w985 -> [_ w999]
              frame False {
              }
              frame True {
                # "User Friendly Input Table"
                # "Command Auto Lookup"
                n725 = call "DIsco_CommList.vi"("Command In"=w999) -> ("Exists?"=w998:bool, "Command Out"=w997:string, "Command Description"=w996:string)  [unwired: 11 in, 1 out]
                n726 = for {
                  N: w1003 -> [_]
                  shift-right: [w1017] -> w1000
                  shift-left: w1002 -> [w1016]
                  tunnel: w1001 -> [w1012]
                  i -> [w1013]
                  n727 = Subtract(x=w1013, y=w1012) -> (x-y=w1011:i32)
                  n728 = Decrement(x=w1011) -> (x-1=w1010:i32)
                  n729 = Format Value(format string="%d", value (0)=w1010) -> (output string=w1014:string)  [unwired: 1 in]
                  n730 = Build Array (concatenate)(w1016, w1014) -> (w1017:string[])
                }
                n731 = case shown="True" w998 {
                  tunnel: w997 -> [w1006 _]
                  tunnel: w996 -> [w1005 _]
                  frame True {
                    n732 = Concatenate Strings(w1006, " : " ("string"), w1005) -> (→"Meaning":string)
                  }
                  frame False {
                    n733 = local write "Meaning"("***INVALID COMMAND***" ("Meaning")) -> ()
                  }
                }
                n734 = local write "Prev Select"(w1004) -> ()
                n735 = property on="Program Edit Table" class="Tbl (strict)"("Row Headers[]"=w1000) -> ()  [unwired: 2 in, 2 out]
              }
            }
          }
          frame #21 {
            # "Activate Pump Routine"
            n736 = case shown="True" "Set Program" {
              frame False {
              }
              frame True {
                n737 = stacked-sequence {
                  frame #0 {
                    n738 = local read "Routine Name"() -> (w1022:string)
                    n739 = local read "Program Edit Table"() -> (w1023:string[][])
                    n740 = local read "Program Selector"() -> (w1024:i32)
                    n741 = call "DIsco_AddProgram.vi"("Program Edit Table"=w1023, "Program Name"=w1022, "Selector in"=w1024) -> ("Program Edit Table 2"=w1020:string[][], "Selector out"=w1025:i32)  [unwired: 7 in]
                    n742 = local write "Run Program"(FALSE ("Run Program")) -> ()
                    n743 = local write "Program Edit Table"(w1020) -> ()
                    n744 = local write "Program Selector"(w1025) -> ()
                  }
                  frame #1 {
                    n745 = global read "DIsco_Globals.vi" "Program Names"() -> (w1028:string[])
                    n746 = local read "Routine Name"() -> (w1027:string)
                    n747 = global read "DIsco_Globals.vi" "Program Stack"() -> (w1029:string[][][])
                    n748 = call "DIsco_SubSelector.vi"("Passing String (Program Name)"=w1027, "Program Names"=w1028, "Program Stack"=w1029) -> ("Selected Program Name"=w1032:string, "Active Program"=w1034:string[][])  [unwired: 7 in]
                    "Running Program" <- w1034
                    n749 = local write "Set Program"(FALSE ("Set Program")) -> ()
                    n750 = property on="Reset" class="Bool (strict)"("Blinking"=FALSE) -> ()  [unwired: 2 in, 2 out]
                    n751 = local write "Active Routine"(w1032) -> ()
                    n752 = local write "Heirarchy"(w1032) -> ()
                    n753 = local write "Step"(0 ("Current\nProgram\nStep")) -> ()
                    n754 = call "DIsco_ParseProgram.vi"("Program Array"=w1034) -> ("Truncated Array"=w1026:string[][])  [unwired: 8 in, 2 out]
                    n755 = global write "DIsco_Globals.vi" "Running Routine"(w1026) -> ()
                    n756 = global write "DIsco_Globals.vi" "Active Program"(w1034) -> ()
                  }
                }
              }
            }
            n757 = local read "Run Program"() -> (→"Program":bool)
          }
        }
        n758 = local read "EXIT"() -> (w620:bool)
        n759 = Wait (ms)(milliseconds to wait=u32 25) -> ()  [unwired: 1 out]
        "EXIT" <- "stop"
      }
      n760 = while {
        shift-right: [w1060] -> _
        shift-left: 0 ("Increment Out") -> [w1057]
        shift-right: [w1059] -> _
        shift-left: u32 0 ("Next Call Out") -> [w1058]
        shift-right: [w1055] -> _
        shift-left: u32 0 ("Next Call Out") -> [w1056]
        stop <- w1054 stop-if-true
        n761 = stacked-sequence {
          seq-local: [w1064 _ _ _ _ _ _ _ _ _ _ _ _ _ _ _ _ _ _ _ _ _ _ _ _ _] -> [_ w1094 w1111 w1134 w1151 _ _ _ _ _ _ _ _ _ _ _ _ _ _ _ _ _ _ w1605 w1629 _]
          seq-local: [w1062 _ _ _ _ _ _ _ _ _ _ _ _ _ _ _ _ _ _ _ _ _ _ _ _ _] -> [_ w1093 _ _ _ _ _ _ _ _ _ _ _ _ _ _ _ _ _ _ _ _ _ _ _ _]
          tunnel: w1058 -> [w1071 _ _ _ _ w1169 w1185 w1206 w1220 w1236 w1254 w1272 w1290 w1306 w1323 w1340 w1354 w1387 w1422 w1446 w1472 _ w1600 _ _ _]
          tunnel: w1057 -> [w1070 _ _ _ _ w1168 w1184 w1205 w1219 w1235 w1253 w1271 w1289 w1305 w1322 w1339 w1353 w1386 w1421 w1445 w1471 _ w1599 _ _ _]
          tunnel: [w1069 _ _ _ _ _ _ _ _ _ _ _ _ _ _ _ _ _ _ _ _ _ _ _ _ _] -> w1060
          tunnel: [w1068 _ _ _ _ _ _ _ _ _ _ _ _ _ _ _ _ _ _ _ _ _ _ _ _ _] -> w1059
          tunnel: w1056 -> [_ _ _ _ _ _ _ _ _ _ _ _ _ _ _ _ _ _ _ _ w1464 _ _ _ _ _]
          tunnel: [_ _ _ _ _ _ _ _ _ _ _ _ _ _ _ _ _ _ _ _ w1466 _ _ _ _ _] -> w1055
          tunnel: [w1061 _ _ _ _ _ _ _ _ _ _ _ _ _ _ _ _ _ _ _ _ _ _ _ _ _] -> w1052
          tunnel: [_ _ _ _ _ w1162 _ _ _ _ _ _ _ _ _ _ _ _ _ _ _ _ _ _ _ _] -> w1051
          tunnel: [_ _ _ _ _ _ w1176 _ _ _ _ _ _ _ _ _ _ _ _ _ _ _ _ _ _ _] -> w1050
          tunnel: [_ _ _ _ _ _ _ w1199 _ _ _ _ _ _ _ _ _ _ _ _ _ _ _ _ _ _] -> w1049
          tunnel: [_ _ _ _ _ _ _ _ w1213 _ _ _ _ _ _ _ _ _ _ _ _ _ _ _ _ _] -> w1048
          tunnel: [_ _ _ _ _ _ _ _ _ w1227 _ _ _ _ _ _ _ _ _ _ _ _ _ _ _ _] -> w1047
          tunnel: [_ _ _ _ _ _ _ _ _ _ w1245 _ _ _ _ _ _ _ _ _ _ _ _ _ _ _] -> w1046
          tunnel: [_ _ _ _ _ _ _ _ _ _ _ w1263 _ _ _ _ _ _ _ _ _ _ _ _ _ _] -> w1045
          tunnel: [_ _ _ _ _ _ _ _ _ _ _ _ w1281 _ _ _ _ _ _ _ _ _ _ _ _ _] -> w1044
          tunnel: [_ _ _ _ _ _ _ _ _ _ _ _ _ w1299 _ _ _ _ _ _ _ _ _ _ _ _] -> w1043
          tunnel: [_ _ _ _ _ _ _ _ _ _ _ _ _ _ w1316 _ _ _ _ _ _ _ _ _ _ _] -> w1042
          tunnel: [_ _ _ _ _ _ _ _ _ _ _ _ _ _ _ w1333 _ _ _ _ _ _ _ _ _ _] -> w1041
          tunnel: [_ _ _ _ _ _ _ _ _ _ _ _ _ _ _ _ w1347 _ _ _ _ _ _ _ _ _] -> w1040
          tunnel: [_ _ _ _ _ _ _ _ _ _ _ _ _ _ _ _ _ w1380 _ _ _ _ _ _ _ _] -> w1039
          tunnel: [_ _ _ _ _ _ _ _ _ _ _ _ _ _ _ _ _ _ w1413 _ _ _ _ _ _ _] -> w1038
          tunnel: [_ _ _ _ _ _ _ _ _ _ _ _ _ _ _ _ _ _ _ w1439 _ _ _ _ _ _] -> w1037
          tunnel: [_ _ _ _ _ _ _ _ _ _ _ _ _ _ _ _ _ _ _ _ w1459 _ _ _ _ _] -> w1036
          frame #0 {
            # "Data Call All Channels"
            n762 = call "DIsco_Call.vi"("Sampling Rate \n(0.001 to 1 Hz)"="Data Call Rate", "Increment In"=w1070, "Next Call In"=w1071, "Enable Next Increment"=TRUE) -> ("Increment Out"=w1069:i32, "Next Call Out"=w1068:u32, "TRUE Aux Time"=→"AUX":bool, "TRUE Call Now"=w1064:bool)  [unwired: 4 in]
            "CALL" <- w1064
            n763 = Tick Count (ms)() -> (millisecond timer value=w1063:u32)
            n764 = case shown="True" w1064 {
              tunnel: [w1073 w1076] -> w1062
              tunnel: w1063 -> [w1073 w1076]
              tunnel: [w1072 w1074] -> w1061
              frame False {
                n765 = local read "COM"() -> (w1072:bool)
              }
              frame True {
                n766 = global read "DIsco_Globals.vi" "Call_List"() -> (w1077:dbl[][])
                n767 = Array Size(array=w1077) -> (size(s)=w1080:i32[])
                n768 = Index Array(array=w1080, index=0) -> (element=w1078:i32)
                n769 = for {
                  N: w1078 -> [_]
                  shift-right: [w1085] -> w1074
                  shift-left: TRUE ("Enable Next Increment") -> [w1081]
                  i -> [w1087]
                  n770 = Equal To 0?(x=w1087) -> (x = 0?=w1089:bool)
                  n771 = case shown="True" w1089 {
                    frame False {
                    }
                    frame True {
                      # "Date and Time"
                      n772 = Format Date/Time String(time format string (%c)="%m/%d/%y %H:%M:%S%2u UTC", UTC format=TRUE) -> (date/time string=→"Date":string)  [unwired: 1 in]
                    }
                  }
                  n773 = call "DIsco_Comms.vi"("DIsco Command"="DIGITAL", "Call Index"=w1087) -> ("Checksum"=w1084:bool)  [unwired: 11 in, 2 out]
                  n774 = call "DIsco_Comms.vi"("DIsco Command"="GET ALL", "Call Index"=w1087) -> ("Checksum"=w1083:bool)  [unwired: 11 in, 2 out]
                  n775 = And(x=w1084, y=w1083) -> (x .and. y?=w1082:bool)
                  n776 = Select(t=w1081, s=w1082, f=w1082) -> (s? t:f=w1085:bool)
                }
              }
            }
          }
          frame #1 {
            # "Calculate Time"
            n777 = case shown="True" w1094 {
              tunnel: w1093 -> [_ w1095]
              frame False {
              }
              frame True {
                n778 = global read "DIsco_Globals.vi" "History_Data"() -> (w1102:dbl[][])
                n779 = Tick Count (ms)() -> (millisecond timer value=w1096:u32)
                n780 = Array Size(array=w1102) -> (size(s)=w1101:i32[])
                n781 = Subtract(x=w1096, y=w1095) -> (x-y=→"Call Execution Time (ms)":u32)
                n782 = Index Array(array=w1101, index=0) -> (element=w1098:i32)
                n783 = Greater Than 0?(x=w1098) -> (x > 0?=w1099:bool)
                n784 = case shown="True" w1099 {
                  frame False {
                    n785 = call "DIsco_SetVar.vi"("NewValue"=0.0, "AccessName"="Time") -> ()  [unwired: 3 in, 1 out]
                  }
                  frame True {
                    n786 = local read "Start Time"() -> (w1105:dbl)
                    n787 = call "GetDate1900.vi"() -> ("current time (1900)"=w1106:dbl)  [unwired: 1 in]
                    n788 = Subtract(x=w1106, y=w1105) -> (x-y=w1110:dbl)
                    n789 = Multiply(x=1440.0, y=w1110) -> (x*y=w1108:dbl)
                    n790 = call "DIsco_SetVar.vi"("NewValue"=w1108, "AccessName"="Time") -> ()  [unwired: 3 in, 1 out]
                  }
                }
              }
            }
          }
          frame #2 {
            # "Update Variable Values"
            n791 = case shown="True" w1111 {
              frame False {
              }
              frame True {
                n792 = global read "DIsco_Globals.vi" "Pump_Status"() -> (w1127:string[][])
                n793 = global read "DIsco_Globals.vi" "Pump_Data"() -> (w1126:dbl[][])
                n794 = global read "DIsco_Globals.vi" "Pump_Data"() -> (w1121:dbl[][])
                n795 = global read "DIsco_Globals.vi" "Pump_Data"() -> (w1118:dbl[][])
                n796 = global read "DIsco_Globals.vi" "Pump_List"() -> (w1133:string[][])
                n797 = Index Array(array=w1126, index (col)=0 ("disabled index (col)")) -> (element=w1125:dbl[])  [unwired: 1 in]
                n798 = Index Array(array=w1121, index (col)=1 ("disabled index (col)")) -> (element=w1122:dbl[])  [unwired: 1 in]
                n799 = Index Array(array=w1118, index (col)=2 ("disabled index (col)")) -> (element=w1117:dbl[])  [unwired: 1 in]
                n800 = Number To Fractional String(number=w1125, precision (6)=i16 0) -> (F-format string=w1115:string[])  [unwired: 2 in]
                n801 = Number To Fractional String(number=w1122, precision (6)=i16 6) -> (F-format string=w1114:string[])  [unwired: 2 in]
                n802 = Number To Fractional String(number=w1117, precision (6)=i16 3) -> (F-format string=w1113:string[])  [unwired: 2 in]
                n803 = call "DIsco_VarAutoUpdate.vi"() -> ()  [unwired: 12 in]
                n804 = Transpose 2D Array(2D array=w1127) -> (transposed array=w1112:string[][])
                n805 = Index Array(array=w1133, index (col)=0 ("disabled index (col)")) -> (element=w1131:string[])  [unwired: 1 in]
                n806 = Build Array (concatenate)(w1131, w1115, w1114, w1113, w1112) -> (w1130:string[][])
                n807 = Transpose 2D Array(2D array=w1130) -> (transposed array=→"Pump Matrix":string[][])
              }
            }
          }
          frame #3 {
            # "Save Data"
            n808 = case shown="True" w1134 {
              frame False {
              }
              frame True {
                n809 = global read "DIsco_Globals.vi" "Pump_Data"() -> (w1144:dbl[][])
                n810 = Array Size(array=w1144) -> (size(s)=w1145:i32[])
                n811 = Index Array(array=w1145, index=0) -> (element=w1137:i32)
                n812 = call "GetDate1900.vi"() -> ("current time (1900)"=w1141:dbl)  [unwired: 1 in]
                n813 = call "DIsco_StatusToComment.vi"() -> ("Status Comment"=w1136:string)  [unwired: 11 in]
                n814 = global read "DIsco_Globals.vi" "History_Data"() -> (w1138:dbl[][])
                n815 = call "DIsco_ExtVarHist.vi"() -> ("Array"=w1135:dbl[])  [unwired: 11 in]
                n816 = Multiply(x=w1137, y=3 ("index")) -> (x*y=w1142:i32)
                n817 = Reshape Array(w1144, w1142) -> (w1140:dbl[])
                n818 = call "Convert to Dynamic Data"("Array"=w1140) -> ("Dynamic Data Type"=w1150:dynamicdata)  [unwired: 3 in]
                n819 = Build Array (concatenate)(w1135, w1138) -> (w1139:dbl[][])
                n820 = global write "DIsco_Globals.vi" "History_Data"(w1139) -> ()
                n821 = Merge Signals(w1141, w1150) -> (w1149:dynamicdata)
                n822 = call "Write To Measurement File"("Signals"=w1149, "Enable"="Enable Data Saving", "Filename"="Filename", "Comment"=w1136) -> ()  [unwired: 13 in, 3 out]
              }
            }
          }
          frame #4 {
            # "Limit Data Length"
            n823 = case shown="True" w1151 {
              frame False {
              }
              frame True {
                w1152 = 10000 ("y")
                n824 = global read "DIsco_Globals.vi" "History_Data"() -> (w1154:dbl[][])
                n825 = Array Size(array=w1154) -> (size(s)=w1157:i32[])
                n826 = Index Array(array=w1157, index=0) -> (element=w1153:i32)
                n827 = Greater?(x=w1153, y=w1152) -> (0:w1155:bool)
                n828 = case shown="True" w1155 {
                  tunnel: w1154 -> [_ w1161]
                  tunnel: w1152 -> [_ w1158]
                  frame False {
                  }
                  frame True {
                    n829 = Array Subset(array=w1161, index (row)=0 ("index"), length (row)=w1158) -> (w1159:dbl[][])  [unwired: 2 in]
                    n830 = global write "DIsco_Globals.vi" "History_Data"(w1159) -> ()
                  }
                }
              }
            }
          }
          frame #5 {
            # "Manual: Stop All Pumps"
            n831 = local read "Data Call Rate"() -> (w1163:dbl)
            n832 = call "DIsco_Call.vi"("Sampling Rate \n(0.001 to 1 Hz)"=w1163, "Increment In"=w1168, "Next Call In"=w1169, "Enable Next Increment"=FALSE) -> ("TRUE Aux Time"=w1165:bool, "TRUE Call Now"=w1167:bool)  [unwired: 4 in, 2 out]
            n833 = local write "CALL"(w1167) -> ()
            n834 = local write "AUX"(w1165) -> ()
            n835 = And(x="Stop Pumps", y=w1165) -> (x .and. y?=w1166:bool)
            n836 = case shown="False" w1166 {
              tunnel: [TRUE ("Checksum") w1172] -> w1162
              frame False {
              }
              frame True {
                n837 = call "DIsco_Comms.vi"("DIsco Command"="STOP ALL") -> ("Checksum"=w1172:bool)  [unwired: 12 in, 2 out]
                n838 = local write "Run Program"(FALSE ("Run Program")) -> ()
                n839 = property on="Stop Pumps" class="Bool (strict)"("Value"=FALSE ("Stop Pumps")) -> ()  [unwired: 2 in, 2 out]
              }
            }
          }
          frame #6 {
            # "Manual: Remote/Internal Control"
            n840 = local read "Remote Indicator"() -> (w1178:bool)
            n841 = local read "Data Call Rate"() -> (w1180:dbl)
            n842 = call "DIsco_Call.vi"("Sampling Rate \n(0.001 to 1 Hz)"=w1180, "Increment In"=w1184, "Next Call In"=w1185, "Enable Next Increment"=FALSE) -> ("TRUE Aux Time"=w1181:bool, "TRUE Call Now"=w1183:bool)  [unwired: 4 in, 2 out]
            n843 = Not Equal?(x=w1178, y="Remote") -> (x != y?=w1179:bool)
            n844 = local write "CALL"(w1183) -> ()
            n845 = local write "AUX"(w1181) -> ()
            n846 = And(x=w1179, y=w1181) -> (x .and. y?=w1182:bool)
            n847 = case shown="False" w1182 {
              tunnel: "Remote" -> [_ w1189]
              tunnel: [TRUE ("Checksum") w1188] -> w1176
              frame False {
              }
              frame True {
                n848 = case shown="True" w1189 {
                  tunnel: [FALSE ("Stop Pumps") TRUE ("Stop Pumps")] -> w1190
                  tunnel: [w1191 w1195] -> w1188
                  frame False {
                    n849 = local read "Pump Index"() -> (w1192:i32)
                    n850 = call "DIsco_Comms.vi"("DIsco Command"="LOCAL", "Pump Index"=w1192) -> ("Checksum"=w1191:bool)  [unwired: 11 in, 2 out]
                  }
                  frame True {
                    n851 = local read "Pump Index"() -> (w1196:i32)
                    n852 = call "DIsco_Comms.vi"("DIsco Command"="REMOTE", "Pump Index"=w1196) -> ("Checksum"=w1195:bool)  [unwired: 11 in, 2 out]
                  }
                }
                "Remote Indicator" <- w1190
              }
            }
          }
          frame #7 {
            # "Manual: Stop Single"
            n853 = local read "Data Call Rate"() -> (w1200:dbl)
            n854 = call "DIsco_Call.vi"("Sampling Rate \n(0.001 to 1 Hz)"=w1200, "Increment In"=w1205, "Next Call In"=w1206, "Enable Next Increment"=FALSE) -> ("TRUE Aux Time"=w1202:bool, "TRUE Call Now"=w1204:bool)  [unwired: 4 in, 2 out]
            n855 = local write "CALL"(w1204) -> ()
            n856 = local write "AUX"(w1202) -> ()
            n857 = And(x="Stop", y=w1202) -> (x .and. y?=w1203:bool)
            n858 = case shown="False" w1203 {
              tunnel: [TRUE ("Checksum") w1209] -> w1199
              frame False {
              }
              frame True {
                n859 = local read "Pump Index"() -> (w1210:i32)
                n860 = local write "Stop"(FALSE ("Stop")) -> ()
                n861 = call "DIsco_Comms.vi"("DIsco Command"="STOP", "Pump Index"=w1210) -> ("Checksum"=w1209:bool)  [unwired: 11 in, 2 out]
              }
            }
          }
          frame #8 {
            # "Manual: Run Single"
            n862 = local read "Data Call Rate"() -> (w1214:dbl)
            n863 = call "DIsco_Call.vi"("Sampling Rate \n(0.001 to 1 Hz)"=w1214, "Increment In"=w1219, "Next Call In"=w1220, "Enable Next Increment"=FALSE) -> ("TRUE Aux Time"=w1216:bool, "TRUE Call Now"=w1218:bool)  [unwired: 4 in, 2 out]
            n864 = local write "CALL"(w1218) -> ()
            n865 = local write "AUX"(w1216) -> ()
            n866 = And(x="Run", y=w1216) -> (x .and. y?=w1217:bool)
            n867 = case shown="False" w1217 {
              tunnel: [TRUE ("Checksum") w1223] -> w1213
              frame False {
              }
              frame True {
                n868 = local read "Pump Index"() -> (w1224:i32)
                n869 = local write "Run"(FALSE ("Run")) -> ()
                n870 = call "DIsco_Comms.vi"("DIsco Command"="RUN", "Pump Index"=w1224) -> ("Checksum"=w1223:bool)  [unwired: 11 in, 2 out]
              }
            }
          }
          frame #9 {
            # "Manual: Set Constant Pressure Mode Single"
            n871 = local read "CP Ind"() -> (w1228:bool)
            n872 = local read "Data Call Rate"() -> (w1231:dbl)
            n873 = call "DIsco_Call.vi"("Sampling Rate \n(0.001 to 1 Hz)"=w1231, "Increment In"=w1235, "Next Call In"=w1236, "Enable Next Increment"=FALSE) -> ("TRUE Aux Time"=w1232:bool, "TRUE Call Now"=w1234:bool)  [unwired: 4 in, 2 out]
            n874 = Not Equal?(x=w1228, y="CP") -> (x != y?=w1230:bool)
            n875 = local write "CALL"(w1234) -> ()
            n876 = local write "AUX"(w1232) -> ()
            n877 = And(x=w1230, y=w1232) -> (x .and. y?=w1233:bool)
            n878 = case shown="False" w1233 {
              tunnel: [TRUE ("Checksum") w1239] -> w1227
              frame False {
              }
              frame True {
                n879 = flat-sequence {
                  tunnel: [w1241] -> w1239
                  frame #0 {
                    n880 = local read "Pump Index"() -> (w1242:i32)
                    n881 = call "DIsco_Comms.vi"("DIsco Command"="CP MODE", "Pump Index"=w1242) -> ("Checksum"=w1241:bool)  [unwired: 11 in, 2 out]
                  }
                  frame #1 {
                    n882 = local write "Fetch"(-1 ("Fetch")) -> ()
                  }
                }
                n883 = local write "CP Ind"(TRUE ("CP Ind")) -> ()
              }
            }
          }
          frame #10 {
            # "Manual: Set Constant Flow Mode Single"
            n884 = local read "Data Call Rate"() -> (w1249:dbl)
            n885 = local read "CF Ind"() -> (w1248:bool)
            n886 = call "DIsco_Call.vi"("Sampling Rate \n(0.001 to 1 Hz)"=w1249, "Increment In"=w1253, "Next Call In"=w1254, "Enable Next Increment"=FALSE) -> ("TRUE Aux Time"=w1250:bool, "TRUE Call Now"=w1252:bool)  [unwired: 4 in, 2 out]
            n887 = Not Equal?(x=w1248, y="CF") -> (x != y?=w1246:bool)
            n888 = local write "CALL"(w1252) -> ()
            n889 = local write "AUX"(w1250) -> ()
            n890 = And(x=w1246, y=w1250) -> (x .and. y?=w1251:bool)
            n891 = case shown="False" w1251 {
              tunnel: [TRUE ("Checksum") w1257] -> w1245
              frame False {
              }
              frame True {
                n892 = flat-sequence {
                  tunnel: [w1259] -> w1257
                  frame #0 {
                    n893 = local read "Pump Index"() -> (w1261:i32)
                    n894 = call "DIsco_Comms.vi"("DIsco Command"="CF MODE", "Pump Index"=w1261) -> ("Checksum"=w1259:bool)  [unwired: 11 in, 2 out]
                  }
                  frame #1 {
                    n895 = local write "Fetch"(-1 ("Fetch")) -> ()
                  }
                }
                n896 = local write "CF Ind"(TRUE ("CF Ind")) -> ()
              }
            }
          }
          frame #11 {
            # "Manual: Set Continuous Pressure Mode"
            n897 = local read "CCP Ind"() -> (w1266:bool)
            n898 = local read "Data Call Rate"() -> (w1267:dbl)
            n899 = call "DIsco_Call.vi"("Sampling Rate \n(0.001 to 1 Hz)"=w1267, "Increment In"=w1271, "Next Call In"=w1272, "Enable Next Increment"=FALSE) -> ("TRUE Aux Time"=w1268:bool, "TRUE Call Now"=w1270:bool)  [unwired: 4 in, 2 out]
            n900 = Not Equal?(x=w1266, y="CCP") -> (x != y?=w1264:bool)
            n901 = local write "CALL"(w1270) -> ()
            n902 = local write "AUX"(w1268) -> ()
            n903 = And(x=w1264, y=w1268) -> (x .and. y?=w1269:bool)
            n904 = case shown="False" w1269 {
              tunnel: [TRUE ("Checksum") w1275] -> w1263
              frame False {
              }
              frame True {
                n905 = flat-sequence {
                  tunnel: [w1277] -> w1275
                  frame #0 {
                    n906 = local read "Pump Index"() -> (w1279:i32)
                    n907 = call "DIsco_Comms.vi"("DIsco Command"="CCP MODE", "Pump Index"=w1279) -> ("Checksum"=w1277:bool)  [unwired: 11 in, 2 out]
                  }
                  frame #1 {
                    n908 = local write "Fetch"(-1 ("Fetch")) -> ()
                  }
                }
                n909 = local write "CCP Ind"(TRUE ("CCP Ind")) -> ()
              }
            }
          }
          frame #12 {
            # "Manual: Set Continuous Flow Mode"
            n910 = local read "Data Call Rate"() -> (w1285:dbl)
            n911 = local read "CCF Ind"() -> (w1284:bool)
            n912 = call "DIsco_Call.vi"("Sampling Rate \n(0.001 to 1 Hz)"=w1285, "Increment In"=w1289, "Next Call In"=w1290, "Enable Next Increment"=FALSE) -> ("TRUE Aux Time"=w1286:bool, "TRUE Call Now"=w1288:bool)  [unwired: 4 in, 2 out]
            n913 = Not Equal?(x=w1284, y="CCF") -> (x != y?=w1282:bool)
            n914 = local write "CALL"(w1288) -> ()
            n915 = local write "AUX"(w1286) -> ()
            n916 = And(x=w1282, y=w1286) -> (x .and. y?=w1287:bool)
            n917 = case shown="False" w1287 {
              tunnel: [TRUE ("Checksum") w1293] -> w1281
              frame False {
              }
              frame True {
                n918 = flat-sequence {
                  tunnel: [w1295] -> w1293
                  frame #0 {
                    n919 = local read "Pump Index"() -> (w1297:i32)
                    n920 = call "DIsco_Comms.vi"("DIsco Command"="CCF MODE", "Pump Index"=w1297) -> ("Checksum"=w1295:bool)  [unwired: 11 in, 2 out]
                  }
                  frame #1 {
                    n921 = local write "Fetch"(-1 ("Fetch")) -> ()
                  }
                }
                n922 = local write "CCF Ind"(TRUE ("CCF Ind")) -> ()
              }
            }
          }
          frame #13 {
            # "Manual: Set Pressure Target"
            n923 = local read "Data Call Rate"() -> (w1301:dbl)
            n924 = call "DIsco_Call.vi"("Sampling Rate \n(0.001 to 1 Hz)"=w1301, "Increment In"=w1305, "Next Call In"=w1306, "Enable Next Increment"=FALSE) -> ("TRUE Aux Time"=w1302:bool, "TRUE Call Now"=w1304:bool)  [unwired: 4 in, 2 out]
            n925 = local write "CALL"(w1304) -> ()
            n926 = local write "AUX"(w1302) -> ()
            n927 = And(x="SetPress", y=w1302) -> (x .and. y?=w1303:bool)
            n928 = case shown="False" w1303 {
              tunnel: [TRUE ("Checksum") w1309] -> w1299
              frame False {
              }
              frame True {
                n929 = local read "Pump Index"() -> (w1313:i32)
                n930 = local write "SetPress"(FALSE ("Run")) -> ()
                n931 = Format Value(format string="%g", value (0)="Pressure Setpoint") -> (output string=w1312:string)  [unwired: 1 in]
                n932 = call "DIsco_Comms.vi"("DIsco Command"="SP=", "Pump Index"=w1313, "DIsco Append"=w1312) -> ("Checksum"=w1309:bool)  [unwired: 10 in, 2 out]
              }
            }
          }
          frame #14 {
            # "Manual: Set Flow Rate Target"
            n933 = local read "Data Call Rate"() -> (w1318:dbl)
            n934 = call "DIsco_Call.vi"("Sampling Rate \n(0.001 to 1 Hz)"=w1318, "Increment In"=w1322, "Next Call In"=w1323, "Enable Next Increment"=FALSE) -> ("TRUE Aux Time"=w1319:bool, "TRUE Call Now"=w1321:bool)  [unwired: 4 in, 2 out]
            n935 = local write "CALL"(w1321) -> ()
            n936 = local write "AUX"(w1319) -> ()
            n937 = And(x="SetFlow", y=w1319) -> (x .and. y?=w1320:bool)
            n938 = case shown="False" w1320 {
              tunnel: [TRUE ("Checksum") w1326] -> w1316
              frame False {
              }
              frame True {
                n939 = local read "Pump Index"() -> (w1328:i32)
                n940 = local write "SetFlow"(FALSE ("Run")) -> ()
                n941 = Format Value(format string="%g", value (0)="Flow Setpoint") -> (output string=w1330:string)  [unwired: 1 in]
                n942 = call "DIsco_Comms.vi"("DIsco Command"="SQ=", "Pump Index"=w1328, "DIsco Append"=w1330) -> ("Checksum"=w1326:bool)  [unwired: 10 in, 2 out]
              }
            }
          }
          frame #15 {
            # "Manual: Zero Pressure"
            n943 = local read "Data Call Rate"() -> (w1335:dbl)
            n944 = call "DIsco_Call.vi"("Sampling Rate \n(0.001 to 1 Hz)"=w1335, "Increment In"=w1339, "Next Call In"=w1340, "Enable Next Increment"=FALSE) -> ("TRUE Aux Time"=w1336:bool, "TRUE Call Now"=w1338:bool)  [unwired: 4 in, 2 out]
            n945 = local write "CALL"(w1338) -> ()
            n946 = local write "AUX"(w1336) -> ()
            n947 = And(x="Zero Pres", y=w1336) -> (x .and. y?=w1337:bool)
            n948 = case shown="False" w1337 {
              tunnel: [TRUE ("Checksum") w1343] -> w1333
              frame False {
              }
              frame True {
                n949 = local read "Pump Index"() -> (w1345:i32)
                n950 = local write "Zero Pres"(FALSE ("Run")) -> ()
                n951 = call "DIsco_Comms.vi"("DIsco Command"="ZERO", "Pump Index"=w1345) -> ("Checksum"=w1343:bool)  [unwired: 11 in, 2 out]
              }
            }
          }
          frame #16 {
            # "Manual: Set Valves"
            n952 = local read "Data Call Rate"() -> (w1349:dbl)
            n953 = call "DIsco_Call.vi"("Sampling Rate \n(0.001 to 1 Hz)"=w1349, "Increment In"=w1353, "Next Call In"=w1354, "Enable Next Increment"=FALSE) -> ("TRUE Aux Time"=w1350:bool, "TRUE Call Now"=w1352:bool)  [unwired: 4 in, 2 out]
            n954 = local write "CALL"(w1352) -> ()
            n955 = local write "AUX"(w1350) -> ()
            n956 = And(x="SetValves", y=w1350) -> (x .and. y?=w1351:bool)
            n957 = case shown="False" w1351 {
              tunnel: [TRUE ("Checksum") w1357] -> w1347
              frame False {
              }
              frame True {
                w1369 = "L"
                w1370 = "H"
                n958 = Select(t=w1370, s="Valve 6", f=w1369) -> (s? t:f=w1363:string)
                n959 = Select(t=w1370, s="Valve 7", f=w1369) -> (s? t:f=w1362:string)
                n960 = Select(t=w1370, s="Valve 8", f=w1369) -> (s? t:f=w1361:string)
                n961 = Select(t=w1370, s="Valve", f=w1369) -> (s? t:f=w1368:string)
                n962 = Select(t=w1370, s="Valve 2", f=w1369) -> (s? t:f=w1367:string)
                n963 = Select(t=w1370, s="Valve 3", f=w1369) -> (s? t:f=w1366:string)
                n964 = Select(t=w1370, s="Valve 4", f=w1369) -> (s? t:f=w1365:string)
                n965 = Select(t=w1370, s="Valve 5", f=w1369) -> (s? t:f=w1364:string)
                n966 = Concatenate Strings(w1368, w1367, w1366, w1365, w1364, w1363, w1362, w1361) -> (w1360:string)
                n967 = property on="SetValves" class="Bool (strict)"("Value"=FALSE ("Run")) -> ()  [unwired: 2 in, 2 out]
                n968 = call "DIsco_Comms.vi"("DIsco Command"="DIGITAL=", "Call Index"="Control ID", "DIsco Append"=w1360) -> ("Checksum"=w1357:bool)  [unwired: 10 in, 2 out]
              }
            }
          }
          frame #17 {
            # "Manual: Set Valve Control Individually"
            n969 = local read "Data Call Rate"() -> (w1382:dbl)
            n970 = call "DIsco_Call.vi"("Sampling Rate \n(0.001 to 1 Hz)"=w1382, "Increment In"=w1386, "Next Call In"=w1387, "Enable Next Increment"=FALSE) -> ("TRUE Aux Time"=w1383:bool, "TRUE Call Now"=w1385:bool)  [unwired: 4 in, 2 out]
            n971 = local write "CALL"(w1385) -> ()
            n972 = local write "AUX"(w1383) -> ()
            n973 = And(x="SetValves 2", y=w1383) -> (x .and. y?=w1384:bool)
            n974 = case shown="True" w1384 {
              tunnel: [TRUE ("Checksum") w1390] -> w1380
              frame False {
              }
              frame True {
                w1402 = "R"
                w1403 = "I"
                n975 = local read "Control ID"() -> (w1391:i32)
                n976 = Select(t=w1403, s="Valve 11", f=w1402) -> (s? t:f=w1396:string)
                n977 = Select(t=w1403, s="Valve 10", f=w1402) -> (s? t:f=w1395:string)
                n978 = Select(t=w1403, s="Valve 9", f=w1402) -> (s? t:f=w1394:string)
                n979 = Select(t=w1403, s="Valve 16", f=w1402) -> (s? t:f=w1401:string)
                n980 = Select(t=w1403, s="Valve 15", f=w1402) -> (s? t:f=w1400:string)
                n981 = Select(t=w1403, s="Valve 14", f=w1402) -> (s? t:f=w1399:string)
                n982 = Select(t=w1403, s="Valve 13", f=w1402) -> (s? t:f=w1398:string)
                n983 = Select(t=w1403, s="Valve 12", f=w1402) -> (s? t:f=w1397:string)
                n984 = Concatenate Strings(w1401, w1400, w1399, w1398, w1397, w1396, w1395, w1394) -> (w1393:string)
                n985 = property on="SetValves 2" class="Bool (strict)"("Value"=FALSE ("Run")) -> ()  [unwired: 2 in, 2 out]
                n986 = call "DIsco_Comms.vi"("DIsco Command"="DIGITAL CTRL=", "Call Index"=w1391, "DIsco Append"=w1393) -> ("Checksum"=w1390:bool)  [unwired: 10 in, 2 out]
              }
            }
          }
          frame #18 {
            # "Manual: Set Remote / Internal valve control"
            n987 = local read "Valve R I"() -> (w1416:bool)
            n988 = local read "Data Call Rate"() -> (w1417:dbl)
            n989 = call "DIsco_Call.vi"("Sampling Rate \n(0.001 to 1 Hz)"=w1417, "Increment In"=w1421, "Next Call In"=w1422, "Enable Next Increment"=FALSE) -> ("TRUE Aux Time"=w1418:bool, "TRUE Call Now"=w1420:bool)  [unwired: 4 in, 2 out]
            n990 = Not Equal?(x=w1416, y="Set Valve Control") -> (x != y?=w1415:bool)
            n991 = local write "CALL"(w1420) -> ()
            n992 = local write "AUX"(w1418) -> ()
            n993 = And(x=w1415, y=w1418) -> (x .and. y?=w1419:bool)
            n994 = case shown="False" w1419 {
              tunnel: "Set Valve Control" -> [_ w1428]
              tunnel: [TRUE ("Checksum") w1425] -> w1413
              frame False {
              }
              frame True {
                n995 = local read "Control ID"() -> (w1427:i32)
                n996 = case shown="True" w1428 {
                  tunnel: w1427 -> [w1430 w1435]
                  tunnel: [FALSE ("Valve R I") TRUE ("Valve R I")] -> w1426
                  tunnel: [w1429 w1434] -> w1425
                  frame False {
                    n997 = call "DIsco_Comms.vi"("DIsco Command"="DIGITAL CTRL=", "Call Index"=w1430, "DIsco Append"="IIIIIIII" ("DIsco_Command")) -> ("Checksum"=w1429:bool)  [unwired: 10 in, 2 out]
                  }
                  frame True {
                    n998 = call "DIsco_Comms.vi"("DIsco Command"="DIGITAL CTRL=", "Call Index"=w1435, "DIsco Append"="RRRRRRRR" ("DIsco_Command")) -> ("Checksum"=w1434:bool)  [unwired: 10 in, 2 out]
                  }
                }
                "Valve R I" <- w1426
              }
            }
          }
          frame #19 {
            # "Manual command execution"
            n999 = local read "Data Call Rate"() -> (w1441:dbl)
            n1000 = call "DIsco_Call.vi"("Sampling Rate \n(0.001 to 1 Hz)"=w1441, "Increment In"=w1445, "Next Call In"=w1446, "Enable Next Increment"=FALSE) -> ("TRUE Aux Time"=w1442:bool, "TRUE Call Now"=w1444:bool)  [unwired: 4 in, 2 out]
            n1001 = local write "CALL"(w1444) -> ()
            n1002 = local write "AUX"(w1442) -> ()
            n1003 = And(x="Manual\nExecute", y=w1442) -> (x .and. y?=w1443:bool)
            n1004 = case shown="False" w1443 {
              tunnel: [TRUE ("Checksum") w1449] -> w1439
              frame False {
              }
              frame True {
                n1005 = local write "Manual\nExecute"(FALSE ("Run")) -> ()
                n1006 = global read "DIsco_Globals.vi" "Comms_List"() -> (w1454:string[][])
                n1007 = local read "Browse"() -> (w1451:i32)
                n1008 = Index Array(array=w1454, index (row)=w1451, index (col)=0 ("disabled index (col)")) -> (element=w1452:string)
                n1009 = call "DIsco_Comms.vi"("DIsco Command"=w1452, "Pump Index"="Pump Index 2", "DIsco Append"="Append") -> ("Reply"=→"Previous Serial Reply":string, "Full Command String"=→"Previous Command":string, "Checksum"=w1449:bool)  [unwired: 10 in]
              }
            }
          }
          frame #20 {
            # "Pump routine execution"
            n1010 = local read "Heirarchy"() -> (w1463:string)
            n1011 = local read "Step"() -> (w1465:i32)
            n1012 = local read "Data Call Rate"() -> (w1467:dbl)
            n1013 = call "DIsco_Call.vi"("Sampling Rate \n(0.001 to 1 Hz)"=w1467, "Increment In"=w1471, "Next Call In"=w1472, "Enable Next Increment"=FALSE) -> ("TRUE Aux Time"=w1468:bool, "TRUE Call Now"=w1470:bool)  [unwired: 4 in, 2 out]
            n1014 = call "DIsco_HoldCheck.vi"("Static Time"=w1464, "Heirarchy"=w1463, "Step"=w1465) -> ("Advance Next = True?"=w1462:bool)  [unwired: 8 in]
            n1015 = local write "CALL"(w1470) -> ()
            n1016 = local write "AUX"(w1468) -> ()
            n1017 = And(x=w1462, y="Run Program") -> (x .and. y?=w1460:bool)
            n1018 = And(x=w1460, y=w1468) -> (x .and. y?=w1469:bool)
            n1019 = case shown="True" w1469 {
              tunnel: [w1478 w1497] -> w1466
              tunnel: w1464 -> [w1479 w1495]
              tunnel: [TRUE ("Checksum") w1496] -> w1459
              frame False {
                # "Check Wait Time"
                n1020 = local read "Run Program"() -> (w1477:bool)
                n1021 = global read "DIsco_Globals.vi" "Running Routine"() -> (w1487:string[][])
                n1022 = local read "Reset"() -> (w1475:bool)
                n1023 = Not(x=w1477) -> (.not. x?=w1476:bool)
                n1024 = Or(x=w1476, y=w1475) -> (x .or. y?=w1474:bool)
                n1025 = local read "Step"() -> (w1485:i32)
                n1026 = case shown="True" w1474 {
                  tunnel: w1479 -> [w1493 _]
                  tunnel: [w1493 w1494] -> w1478
                  frame False {
                  }
                  frame True {
                    n1027 = Tick Count (ms)() -> (millisecond timer value=w1494:u32)
                  }
                }
                n1028 = Index Array(array=w1487, index (row)=w1485, index (col)=2 ("disabled index (col)")) -> (element=w1488:string)
                n1029 = Tick Count (ms)() -> (millisecond timer value=w1491:u32)
                n1030 = Scan Value(string=w1488, format string="%d", default (0 dbl)=0) -> (value=w1483:i32)  [unwired: 1 out]
                n1031 = Subtract(x=w1491, y=w1478) -> (x-y=w1484:u32)
                n1032 = Subtract(x=w1483, y=w1484) -> (x-y=w1482:u32)
                n1033 = Divide(x=w1482, y=1000.0 ("Data Call Rate")) -> (x/y=w1480:dbl)
                n1034 = local write "Countdown"(w1480) -> ()
              }
              frame True {
                n1035 = stacked-sequence {
                  tunnel: [_ w1512 _ _ _ _ _] -> w1497
                  tunnel: [w1499 _ _ _ _ _ _] -> w1496
                  tunnel: w1495 -> [_ _ _ w1532 _ _ _]
                  frame #0 {
                    # "Operate Step"
                    n1036 = global read "DIsco_Globals.vi" "Running Routine"() -> (w1504:string[][])
                    n1037 = local read "Step"() -> (w1500:i32)
                    n1038 = call "DIsco_ParseProgram.vi"("Program Array"=w1504) -> ("Numeric Array"=w1503:dbl[][])  [unwired: 8 in, 2 out]
                    n1039 = Index Array(array=w1504, index (row)=w1500, index (col)=3 ("disabled index (col)")) -> (element=w1506:string)
                    n1040 = Index Array(array=w1504, index (row)=w1500, index (col)=0 ("disabled index (col)")) -> (element=w1508:string)
                    n1041 = Index Array(array=w1503, index (row)=w1500, index (col)=1 ("disabled index (col)")) -> (element=w1502:dbl)
                    n1042 = call "DIsco_PassVarValue.vi"("PASS IN"=w1506) -> ("PASS OUT"=w1498:string)
                    n1043 = local write "Passing String"(w1498) -> ()
                    n1044 = To Long Integer(number=w1502) -> (32bit integer=w1501:i32)
                    n1045 = call "DIsco_Comms.vi"("DIsco Command"=w1508, "Pump Index"=w1501, "DIsco Append"=w1498) -> ("Reply"=w1510:string, "Checksum"=w1499:bool)  [unwired: 10 in, 1 out]
                    n1046 = global write "DIsco_Globals.vi" "Return_String"(w1510) -> ()
                    n1047 = case shown="False" w1499 {
                      tunnel: w1499 -> [w1511 _]
                      frame False {
                        n1048 = local write "ERR"(w1511) -> ()
                      }
                      frame True {
                      }
                    }
                  }
                  frame #1 {
                    # "Initialize Wait Timer"
                    n1049 = Tick Count (ms)() -> (millisecond timer value=w1512:u32)
                  }
                  frame #2 {
                    # "Increment Program Step"
                    n1050 = global read "DIsco_Globals.vi" "Running Routine"() -> (w1513:string[][])
                    n1051 = local read "Step"() -> (w1515:i32)
                    n1052 = Array Size(array=w1513) -> (size(s)=w1518:i32[])
                    n1053 = Index Array(array=w1518, index=0) -> (element=w1516:i32)
                    n1054 = Less?(x=w1515, y=w1516) -> (x < y?=w1514:bool)
                    n1055 = case shown="True" w1514 {
                      tunnel: w1515 -> [_ w1520]
                      frame False {
                      }
                      frame True {
                        n1056 = Increment(x=w1520) -> (x+1=w1519:i32)
                        n1057 = local write "Step"(w1519) -> ()
                      }
                    }
                  }
                  frame #3 {
                    # "Check Wait Time"
                    # "Output Program Step and Wait Clock"
                    n1058 = global read "DIsco_Globals.vi" "Running Routine"() -> (w1528:string[][])
                    n1059 = Tick Count (ms)() -> (millisecond timer value=w1533:u32)
                    n1060 = local read "Step"() -> (w1526:i32)
                    "Step" <- w1526
                    n1061 = Subtract(x=w1533, y=w1532) -> (x-y=w1525:u32)
                    n1062 = Index Array(array=w1528, index (row)=w1526, index (col)=2 ("disabled index (col)")) -> (element=w1529:string)
                    n1063 = Scan Value(string=w1529, format string="%d", default (0 dbl)=0) -> (value=w1524:i32)  [unwired: 1 out]
                    n1064 = Subtract(x=w1524, y=w1525) -> (x-y=w1523:u32)
                    n1065 = Divide(x=w1523, y=1000.0 ("Data Call Rate")) -> (x/y=→"Countdown":dbl)
                  }
                  frame #4 {
                    # "Program Subsub"
                    n1066 = global read "DIsco_Globals.vi" "Program Names"() -> (w1536:string[])
                    n1067 = local read "Passing String"() -> (w1542:string)
                    n1068 = global read "DIsco_Globals.vi" "Program Stack"() -> (w1538:string[][][])
                    n1069 = global read "DIsco_Globals.vi" "Active Program"() -> (w1537:string[][])
                    n1070 = global read "DIsco_Globals.vi" "Return_String"() -> (w1539:string)
                    n1071 = local read "Heirarchy"() -> (w1543:string)
                    n1072 = local read "Step"() -> (w1541:i32)
                    n1073 = local read "Active Routine"() -> (w1540:string)
                    n1074 = call "DIsco_SubSub.vi"("Heirarchy In"=w1543, "Passing String (Name of New Program)"=w1542, "Step Count In"=w1541, "Program Stack"=w1538, "Active Program In"=w1537, "Program Names"=w1536, "DASNET Pass"=w1539, "Selected Program In"=w1540) -> ("Heirarchy Out"=w1547:string, "Active Program Out"=w1535:string[][], "Selected Program Name"=w1546:string, "Step Count Out"=w1545:u32, "Errors"=w1544:string)  [unwired: 7 in]
                    n1075 = call "DIsco_ParseProgram.vi"("Program Array"=w1535) -> ("Truncated Array"=w1534:string[][])  [unwired: 8 in, 2 out]
                    n1076 = global write "DIsco_Globals.vi" "Running Routine"(w1534) -> ()
                    n1077 = global write "DIsco_Globals.vi" "Active Program"(w1535) -> ()
                    n1078 = local write "Active Routine"(w1546) -> ()
                    n1079 = local write "Program Errors"(w1544) -> ()
                    n1080 = local write "Heirarchy"(w1547) -> ()
                    n1081 = local write "Step"(w1545) -> ()
                  }
                  frame #5 {
                    # "Check for Conditional"
                    n1082 = global read "DIsco_Globals.vi" "Return_String"() -> (w1548:string)
                    n1083 = String Subset(string=w1548, offset (0)=0, length (rest)=1 ("length (rest)")) -> (substring=w1551:string)
                    n1084 = Equal?(x="@", y=w1551) -> (x = y?=w1549:bool)
                    n1085 = case shown="True" w1549 {
                      tunnel: w1548 -> [_ w1559]
                      frame False {
                        # "Buisness as Usual"
                      }
                      frame True {
                        n1086 = String Subset(string=w1559, offset (0)=1) -> (substring=w1557:string)  [unwired: 1 in]
                        n1087 = local read "Step"() -> (w1555:i32)
                        n1088 = Scan Value(string=w1557, format string="%d") -> (value=w1560:dbl)  [unwired: 1 in, 1 out]
                        n1089 = To Long Integer(number=w1560) -> (32bit integer=w1556:i32)
                        n1090 = Add(x=w1556, y=w1555) -> (x+y=w1554:i32)
                        n1091 = local write "Step"(w1554) -> ()
                      }
                    }
                  }
                  frame #6 {
                    # "Prevent premature exit when \nprograms have equal length"
                    # "Exit at Program End"
                    n1092 = local read "Heirarchy"() -> (w1565:string)
                    n1093 = Search and Replace String(input string=w1565, search string="\\") -> (number of replacements=w1563:i32)  [unwired: 6 in, 3 out]
                    n1094 = Greater Than 0?(x=w1563) -> (x > 0?=w1562:bool)
                    n1095 = case shown="False" w1562 {
                      tunnel: [w1573 TRUE] -> w1566
                      frame False {
                        n1096 = global read "DIsco_Globals.vi" "Running Routine"() -> (w1569:string[][])
                        n1097 = local read "Step"() -> (w1574:i32)
                        n1098 = Array Size(array=w1569) -> (size(s)=w1572:i32[])
                        n1099 = Index Array(array=w1572, index=0) -> (element=w1570:i32)
                        n1100 = Less?(x=w1574, y=w1570) -> (x < y?=w1573:bool)
                      }
                      frame True {
                      }
                    }
                    n1101 = case shown="False" w1566 {
                      frame False {
                        n1102 = property on="Run Program" class="Bool (strict)"("Value"=FALSE ("Run Program")) -> ()  [unwired: 2 in, 2 out]
                        n1103 = local write "Reset"(TRUE ("Reset")) -> ()
                      }
                      frame True {
                      }
                    }
                  }
                }
              }
            }
          }
          frame #21 {
            # "Update variables table"
            n1104 = global read "DIsco_Globals.vi" "V_Names"() -> (w1582:string[])
            n1105 = global read "DIsco_Globals.vi" "V_Values"() -> (w1581:dbl[])
            n1106 = Array Size(array=w1581) -> (size(s)=w1576:i32)
            n1107 = for {
              N: w1576 -> [_]
              shift-right: [w1591] -> w1580
              shift-left: string[][] [] ("Table Control") -> [w1590]
              tunnel: w1581 -> [w1593] mode=indexing
              shift-right: [w1588] -> w1578
              shift-left: string[] [] ("V_Names") -> [w1586]
              tunnel: w1582 -> [w1584] mode=indexing
              i -> [w1589]
              n1108 = Number To Exponential String(number=w1593, precision (6)=i16 6) -> (E-format string=w1585:string)  [unwired: 2 in]
              n1109 = Number To Decimal String(number=w1589) -> (decimal integer string=w1587:string)  [unwired: 1 in]
              n1110 = Build Array (concatenate)(w1586, w1587) -> (w1588:string[])
              n1111 = Build Array(w1584, w1585) -> (w1583:string[])
              n1112 = Build Array (concatenate)(w1590, w1583) -> (w1591:string[][])
            }
            "Table Control" <- w1580
            n1113 = property on="Table Control" class="Tbl (strict)"("Row Headers[]"=w1578) -> ()  [unwired: 2 in, 2 out]
          }
          frame #22 {
            # "Acquire external data"
            n1114 = local read "Data Call Rate"() -> (w1595:dbl)
            n1115 = call "DIsco_Call.vi"("Sampling Rate \n(0.001 to 1 Hz)"=w1595, "Increment In"=w1599, "Next Call In"=w1600, "Enable Next Increment"=FALSE) -> ("TRUE Aux Time"=w1596:bool, "TRUE Call Now"=w1598:bool)  [unwired: 4 in, 2 out]
            n1116 = local write "CALL"(w1598) -> ()
            n1117 = local write "AUX"(w1596) -> ()
            n1118 = And(x="Import", y=w1596) -> (x .and. y?=w1597:bool)
            n1119 = case shown="True" w1597 {
              frame False {
              }
              frame True {
                n1120 = local write "Import"(FALSE ("Import")) -> ()
                n1121 = call "DIsco_Import.vi"("External File Path"="External File Path") -> ("Array"=→"External Data":dbl[][])  [unwired: 10 in]
              }
            }
          }
          frame #23 {
            # "Plot data"
            n1122 = case shown="True" w1605 {
              frame False {
              }
              frame True {
                n1123 = local read "Min_Y 3"() -> (w1621:dbl)
                n1124 = local read "Max_Y 3"() -> (w1623:dbl)
                n1125 = call "DIsco_PlotSelect.vi"("Variable"="X") -> ("Index"=w1606:i32)  [unwired: 10 in]
                n1126 = call "DIsco_PlotSelect.vi"("Variable"="Y1") -> ("Index"=w1618:i32)  [unwired: 10 in]
                n1127 = call "DIsco_PlotSelect.vi"("Variable"="Y2") -> ("Index"=w1608:i32)  [unwired: 10 in]
                n1128 = call "DIsco_PlotSelect.vi"("Variable"="Y3") -> ("Index"=w1609:i32)  [unwired: 10 in]
                n1129 = call "DIsco_PlotSelect.vi"("Variable"="Y4") -> ("Index"=w1610:i32)  [unwired: 10 in]
                n1130 = call "DIsco_PlotSelect.vi"("Variable"="Y5") -> ("Index"=w1611:i32)  [unwired: 10 in]
                n1131 = call "DIsco_PlotSelect.vi"("Variable"="Y6") -> ("Index"=w1612:i32)  [unwired: 10 in]
                n1132 = property on="Plot1 3" class="XYGraph (strict)"("YScale.Minimum"=w1621) -> ()  [unwired: 2 in, 2 out]
                n1133 = property on="Plot1 3" class="XYGraph (strict)"("YScale.Maximum"=w1623) -> ()  [unwired: 2 in, 2 out]
                n1134 = call "DIsco_Plot.vi"("Index_X"=w1606, "Index_Y1"=w1618, "Index_Y2"=w1608, "Index_logY1"=w1611, "Index_logY2"=w1612, "Index_Y3"=w1609, "Index_Y4"=w1610, "Num_Pts"="Num Points 3", "Max_Y"="Max_Y 3", "Max_logY"="Max Log", "Min_Y"="Min_Y 3", "Min_logY"="Min Log") -> ("XY Graph"=→"Plot1 3":cluster{"X":dbl[], "Y":dbl[]}[], "Scaling Relationship"=→"Scaling Relationship 3":string)  [unwired: 14 in]
              }
            }
          }
          frame #24 {
            # "Update history table"
            n1135 = case shown="True" w1629 {
              frame False {
              }
              frame True {
                n1136 = global read "DIsco_Globals.vi" "History_Headers"() -> (w1632:string[])
                n1137 = global read "DIsco_Globals.vi" "History_Data"() -> (w1636:dbl[][])
                n1138 = Array Size(array=w1632) -> (size(s)=w1633:i32)
                n1139 = for {
                  N: w1633 -> [_]
                  tunnel: w1632 -> [w1639] mode=indexing
                  shift-right: [w1642] -> w1630
                  shift-left: string[] [] ("Column Header Strings[]") -> [w1643]
                  i -> [w1641]
                  n1140 = Number To Decimal String(number=w1641) -> (decimal integer string=w1640:string)  [unwired: 1 in]
                  n1141 = Concatenate Strings(w1640, ": " ("string"), w1639) -> (w1638:string)
                  n1142 = Build Array (concatenate)(w1643, w1638) -> (w1642:string[])
                }
                n1143 = Number To Exponential String(number=w1636, precision (6)=i16 2) -> (E-format string=→"Recorded Data":string[][])  [unwired: 2 in]
                n1144 = property on="Recorded Data" class="Tbl (strict)"("Column Headers[]"=w1630) -> ()  [unwired: 2 in, 2 out]
              }
            }
          }
          frame #25 {
            # "Display pump data"
            n1145 = global read "DIsco_Globals.vi" "Pump_Status"() -> (w1670:string[][])
            n1146 = global read "DIsco_Globals.vi" "Pump_Limits"() -> (w1657:dbl[][])
            n1147 = global read "DIsco_Globals.vi" "Pump_Data"() -> (w1650:dbl[][])
            n1148 = global read "DIsco_Globals.vi" "Pump_Data"() -> (w1652:dbl[][])
            n1149 = global read "DIsco_Globals.vi" "Pump_Data"() -> (w1655:dbl[][])
            n1150 = call "DIsco_PumpListParse.vi"("Pump Index In"="Pump Index") -> ("Pump Type"=→"Pump Type":string, "Call Index"=→"Call ID":i32, "Pump Index Out"=w1671:i32, "Pump Name"=→"Name of Selected Pump":string, "Pump Letter"=→"Letter":string)  [unwired: 6 in, 4 out]
            n1151 = Index Array(array=w1670, index (row)=w1671) -> (element=w1646:string[])  [unwired: 1 in]
            n1152 = Index Array(array=w1650, index (row)="Pump Index", index (col)=0 ("disabled index (col)")) -> (element=→"P Active":dbl)
            n1153 = Index Array(array=w1652, index (row)="Pump Index", index (col)=1 ("disabled index (col)")) -> (element=→"F Active":dbl)
            n1154 = Index Array(array=w1655, index (row)="Pump Index", index (col)=2 ("disabled index (col)")) -> (element=w1660:dbl)
            "V Active" <- w1660
            n1155 = Index Array(array=w1657, index (row)="Pump Index", index (col)=5 ("disabled index (col)")) -> (element=w1659:dbl)
            n1156 = call "Parse_Status.vi"("Abbr Status"=w1646) -> ("Full Status"=→"Status":string[])  [unwired: 10 in]
            n1157 = Index Array(array=w1646, index=1) -> (element=w1644:string)
            n1158 = Divide(x=w1660, y=w1659) -> (x/y=w1664:dbl)
            n1159 = Multiply(x=w1664, y=100.0) -> (x*y=w1662:dbl)
            n1160 = Subtract(x=100.0, y=w1662) -> (x-y=→"Vol %":dbl)
            n1161 = case shown="\"L\", Default" w1644 {
              frame "L", Default {
                w1672 = T2."Disabled and Grayed Out" ("Disabled")
                n1162 = property on="Zero Pres" class="Bool (strict)"("DisabledEnum"=w1672) -> ()  [unwired: 2 in, 2 out]
                n1163 = property on="Run" class="Bool (strict)"("DisabledEnum"=w1672) -> ()  [unwired: 2 in, 2 out]
                n1164 = property on="Stop" class="Bool (strict)"("DisabledEnum"=w1672) -> ()  [unwired: 2 in, 2 out]
                n1165 = local write "Remote Indicator"(FALSE) -> ()
                n1166 = property on="SetPress" class="Bool (strict)"("DisabledEnum"=w1672) -> ()  [unwired: 2 in, 2 out]
                n1167 = property on="SetFlow" class="Bool (strict)"("DisabledEnum"=w1672) -> ()  [unwired: 2 in, 2 out]
              }
              frame "R" {
                w1674 = T2."Enabled" ("Disabled")
                n1168 = property on="Zero Pres" class="Bool (strict)"("DisabledEnum"=w1674) -> ()  [unwired: 2 in, 2 out]
                n1169 = property on="Run" class="Bool (strict)"("DisabledEnum"=w1674) -> ()  [unwired: 2 in, 2 out]
                n1170 = property on="Stop" class="Bool (strict)"("DisabledEnum"=w1674) -> ()  [unwired: 2 in, 2 out]
                n1171 = local write "Remote Indicator"(TRUE) -> ()
                n1172 = property on="SetPress" class="Bool (strict)"("DisabledEnum"=w1674) -> ()  [unwired: 2 in, 2 out]
                n1173 = property on="SetFlow" class="Bool (strict)"("DisabledEnum"=w1674) -> ()  [unwired: 2 in, 2 out]
              }
            }
          }
        }
        n1174 = Compound Arithmetic op=AND(w1052, w1051, w1050, w1049, w1048, w1047, w1046, w1045, w1044, w1043, w1042, w1041, w1040, w1039, w1038, w1037, w1036) -> (w1035:bool)
        n1175 = local write "COM"(w1035) -> ()
        n1176 = local read "EXIT"() -> (w1054:bool)
        n1177 = Wait (ms)(milliseconds to wait=u32 5) -> ()  [unwired: 1 out]
      }
    }
    frame #2 {
      # "Save Settings"
      # "Final Commands"
      # "Close Program"
      n1178 = case shown="False" "Stop Pumps on Exit" {
        frame True {
          n1179 = global read "DIsco_Globals.vi" "Call_List"() -> (w1710:dbl[][])
          n1180 = Array Size(array=w1710) -> (size(s)=w1709:i32[])
          n1181 = Index Array(array=w1709, index=0) -> (element=w1707:i32)
          n1182 = stacked-sequence {
            tunnel: w1707 -> [w1711]
            frame #0 {
              n1183 = for {
                N: w1711 -> [_]
                i -> [w1712]
                n1184 = stacked-sequence {
                  tunnel: w1712 -> [w1713 w1715]
                  frame #0 {
                    n1185 = call "DIsco_Comms.vi"("DIsco Command"="CLEAR", "Call Index"=w1713) -> ()  [unwired: 11 in, 3 out]
                  }
                  frame #1 {
                    n1186 = call "DIsco_Comms.vi"("DIsco Command"="LOCAL", "Call Index"=w1715) -> ()  [unwired: 11 in, 3 out]
                  }
                }
              }
            }
          }
        }
        frame False {
        }
      }
      n1187 = local read "Log Commands"() -> (w1700:bool)
      n1188 = local read "Num Points 3"() -> (w1692:i32)
      n1189 = local read "Stop Pumps on Exit"() -> (w1695:bool)
      n1190 = local read "Min Log"() -> (w1688:dbl)
      n1191 = local read "Min_Y 3"() -> (w1690:dbl)
      n1192 = local read "Max Log"() -> (w1689:dbl)
      n1193 = local read "Max_Y 3"() -> (w1691:dbl)
      n1194 = local read "Data Call Rate"() -> (w1693:dbl)
      n1195 = local read "Ask_Auto"() -> (w1699:bool)
      n1196 = local read "X"() -> (w1676:string)
      n1197 = local read "Y1"() -> (w1677:string)
      n1198 = local read "Y2"() -> (w1678:string)
      n1199 = local read "Y3"() -> (w1679:string)
      n1200 = local read "Y4"() -> (w1680:string)
      n1201 = local read "Y5"() -> (w1681:string)
      n1202 = local read "Y6"() -> (w1682:string)
      n1203 = Boolean To (0,1)(Boolean=w1699) -> (0, 1=w1698:i16)
      n1204 = Boolean To (0,1)(Boolean=w1700) -> (0, 1=w1697:i16)
      n1205 = Boolean To (0,1)(Boolean=w1695) -> (0, 1=w1696:i16)
      n1206 = Format Value(format string="%g", value (0)=w1693) -> (output string=w1701:string)  [unwired: 1 in]
      n1207 = Format Value(value (0)=w1696) -> (output string=w1702:string)  [unwired: 2 in]
      n1208 = Format Value(value (0)=w1698) -> (output string=w1703:string)  [unwired: 2 in]
      n1209 = Format Value(value (0)=w1697) -> (output string=w1704:string)  [unwired: 2 in]
      n1210 = Format Value(value (0)=w1692) -> (output string=w1687:string)  [unwired: 2 in]
      n1211 = Format Value(value (0)=w1691) -> (output string=w1686:string)  [unwired: 2 in]
      n1212 = Format Value(value (0)=w1690) -> (output string=w1685:string)  [unwired: 2 in]
      n1213 = Format Value(value (0)=w1689) -> (output string=w1684:string)  [unwired: 2 in]
      n1214 = Format Value(value (0)=w1688) -> (output string=w1683:string)  [unwired: 2 in]
      n1215 = Build Array(w1701, w1702, w1703, w1704, w1676, w1677, w1678, w1679, w1680, w1681, w1682, w1687, w1686, w1685, w1684, w1683) -> (w1705:string[])
      n1216 = call "DIsco_SaveAll.vi"("Array"=w1705) -> ()  [unwired: 11 in]
    }
  }
